vi "WAM-PROD_Sequencer.vi"() -> ()   [LabVIEW 2018]
uses:
  <vilib>/Utility/miscctls.llb/LVPositionTypeDef.ctl
  <vilib>/Utility/miscctls.llb/LVPointTypeDef.ctl
  Labview Utilities/Load and Save Controls_LV2009/RWC_Actions.ctl
  Initialize References/Sequence Globals.vi
  Infrastructure/Test Parameter Globals_1.0.0.vi
  Automated Tests/Tetra WAM/Tetra_Globals.vi
  Infrastructure/Test Result File Name Global.vi
  Initialize References/Station References Global.vi
  <vilib>/Utility/file.llb/Read Delimited Spreadsheet (string).vi
  <vilib>/Utility/file.llb/Write Delimited Spreadsheet (string).vi
panel:
  out "Results Archive File (Location on server)":path=path "C:/RageATE Results/REV-C_P-WAM_TX-ATTEN/2_12_2025/REV-C_P-WAM_TX-ATTEN_SN_WAM-000442_2309_021225-161452.csv" caption="Results Archive File \n(Location on server)"
  out "Seq Start Time":string
  out "Seq End Time":string
  out "Total Test Time":string="0.000"
  in  "User Prompt for SN (T)":bool=TRUE
  out "App Path":string="<dev mode>"
  out "FirstCall(t)":bool
  out "Inst_vi":path=path "C:/RageATE/Automated Tests/Tetra WAM/PRODUCTION/prod test vis/Tetra_PROD_Instruments.vi"
  out "Eng_NumTests":bool[](array[boolean])=[TRUE, TRUE, TRUE, TRUE, TRUE, TRUE, TRUE, TRUE]
  out "vis to run":path[](array[path])=[path "C:/RageATE/Automated Tests/Tetra WAM/PRODUCTION/prod test vis/Tetra_PROD_Instruments.vi", path "C:/RageATE/Infrastructure/GetLoopParameters_16.0.0.0.vi", path "C:/RageATE/Infrastructure/SystemTestIterator_4.3.0.0.vi", path "", path "", path "", path "", path ""]
  out "run?":bool=TRUE
  out "Stop Testing":bool
  out "Array":string[](array[string])=["C:\\RageATE\\Automated Tests\\Tetra WAM\\PRODUCTION\\prod test vis\\Tetra_PROD_Instruments.vi", "C:\\RageATE\\Infrastructure\\GetLoopParameters_16.0.0.0.vi", "C:\\RageATE\\Infrastructure\\SystemTestIterator_4.3.0.0.vi", "", "", "", "", ""]
  out "VI Name":string="WAM-PROD_Sequencer3.vi"
  out "VI Path":path=path "C:/RageATE/Projects/WAM"
  out "db_out_str":string="REV-C_TETRA_TX-ATTEN database id: 5875\r\nMoved REV-C_TETRA_TX-ATTEN_SN_WAM-000412_2248_030323-101631.csv to Synology Drive\r\nSUCCESS\r\nREV-C_TETRA_TX-PROD database id: 5876\r\nMoved REV-C_TETRA_TX-PROD_SN_WAM-000412_2248_030323-101718.csv to Synology Drive\r\nSUCCESS\r\nMoved REV-C_TETRA_RX-PROD_SN_WAM-000412_2248_030323-103734_RxCaptureFiles.zip to Synology Drive\r\nREV-C_TETRA_RX-PROD database id: 5877\r\nMoved REV-C_TETRA_RX-PROD_SN_WAM-000412_2248_030323-103734.csv to Synology Drive\r\nSUCCESS\r\nMoved WAM-C_BOUNCE_SN_WAM-000412_2248_030323-111048_Iq.csv to Synology Drive\r\nWAM-C_BOUNCE database id: 1300\r\nMoved WAM-C_BOUNCE_SN_WAM-000412_2248_030323-111048.csv to Synology Drive\r\nSUCCESS\r\n"
  out "syn_error?(t)":bool
  out "ID":string[](array[string])=["5875", "5876", "5877", "1300"]
  out "UserBCPopup_ref_out":refnum<vi>
  out "user_vi_ref":refnum<vi>
  out "EmpID(str)":string
  in  "LogFilePath":path=path "C:/RageATE Results"
  out "ABORT AT SN SCAN(T)":bool caption="OK"
  out "pw":string="RaGE_062218!"
  out "TestsArray":path[](array[path])=[path "C:/Users/ThomasWattson/OneDrive - Rage Systems/Documents - Tetra/Test Docs/Test Results/PWAM/Test Files/P-WAM-C_TX-ATTEN_Parameters.tst", path "C:/Users/ThomasWattson/OneDrive - Rage Systems/Documents - Tetra/Test Docs/Test Results/PWAM/Test Files/P-WAM-C_RX-PROD_Parameters.tst", path "C:/Users/ThomasWattson/OneDrive - Rage Systems/Documents - Tetra/Test Docs/Test Results/PWAM/Test Files/P-WAM-C_BOUNCE.tst", path "C:/Users/ThomasWattson/OneDrive - Rage Systems/Documents - Tetra/Test Docs/Test Results/PWAM/Test Files/P-WAM-C_TX-PROD_10MHZ_Parameters.tst"]
  out "result files array":path[](array[path])
  out "viRefs":refnum<vi>[](array[refnum])
  out "TestBench_ID":string="WAM_PROD_TEST-1"
  out "current time":timestamp=timestamp(3822239814.3112698 s since 1904-01-01)
  out "Array Element.Value":variant=variant(bool TRUE)
  out "TestResultLink":string="C:\\RageATE Results\\REV-C_P-WAM_TX-ATTEN\\2_12_2025\\REV-C_P-WAM_TX-ATTEN_SN_WAM-000442_2309_021225-161452.csv"
  out "BarCodeInfo":string="#RaGE Systems\r\n#Prod_Name: Wideband Antenna Module\r\n#Rage_PN: 5083561\r\n#Revision: C.08\r\n#LotID: 2309\r\n#MSN: WAM-000442\r\n#ESN: 0x00003A0E2EA5\r\n"
  in  "TabControl":T1(tab)
  in  "Load Tests":bool
  out "FileVersion":string="<dev mode>"
  out "LegalCopyright":string="<dev mode>"
  out "FileDescription":string="<dev mode>"
  out "SW Build":string="<dev mode>"
  in  "SILENCE SAFETY BUZZER":bool
  out "PostProcessMesssage":string
  in  "Test Resolution":bool=TRUE
  in  "Run All Tests (T)":bool=TRUE caption="Place entry into test log"
  in  "Run WAM BOUNCE (T)":bool=TRUE caption="Place entry into test log"
  in  "Run WAM RX (T)":bool=TRUE caption="Place entry into test log"
  in  "Run WAM TX (T)":bool=TRUE caption="Place entry into test log"
  in  "Run WAM-C Atten (t)":bool=TRUE caption="Place entry into test log"
  in  "START TESTING":bool
  out "Test Run 2":string="!!! CHECK EMPLOYEE ID BADGE! ,  Press START to Begin Testing" caption="Running Test: C:\\RageATE\\Automated Tests\\Tetra WAM\\DVT\\Tetra_RX-DVT_Parameters-Quick.tst 1 of 50"
  in  "STOP TESTING":bool
  out "PASS":bool=TRUE
  out "-ssid":string="02122025160254"
  in  "Require System Standard (T)":bool=TRUE caption="BarCoded SN Entry"
  in  "Run Final Test Result":bool=TRUE
  in  "WAM_Bar_Code_Read":bool=TRUE caption="BarCoded SN Entry"
  out "Stop Sequencer":bool
  out "Test Results File Name (Local computer,Automatically generated)":path=path "C:/RageATE Results/REV-C_P-WAM_TX-ATTEN/2_12_2025/REV-C_P-WAM_TX-ATTEN_SN_WAM-000442_2309_021225-161452.csv"
  in  "Open output file\n when test done":bool caption="Open result file automatically upon completion of each test"
  in  "PLace a result file\n copy on server(T)":bool caption="Put a copy of the result file on the server"
  in  "Recipient Email Address (use; to separate addresses)":string="rickq@ragesystems.com"
  in  "Send email notification":bool caption="Send email notification when each test is completed"
  in  "Send as attachment":bool caption="Send result file as an email attachment (if unchecked the location of the result file will be sent)"
  in  "Generate a log file entry for this test":bool=TRUE caption="Place entry into test log"
  in  "Tests Path_Eng":path[](array[path])=[path "C:/RageATE-Tetra/Automated Tests/Tetra WAM/PRODUCTION/setup files/WAM-LC_TX_Parameters -FoilTopCover.tst", path "C:/RageATE-Tetra/Automated Tests/Tetra WAM/PRODUCTION/setup files/WAM-LC_TX_BPF-1_Parameters.tst", path "C:/Users/ThomasWattson/OneDrive - Rage Systems/Documents - Tetra/Test Docs/Test Results/PWAM/Test Files/P-WAM-C_BOUNCE.tst", path "C:/Users/ThomasWattson/OneDrive - Rage Systems/Documents - Tetra/Test Docs/Test Results/PWAM/Test Files/P-WAM-C_TX-PROD_10MHZ_Parameters.tst", path "C:/RageATE/Automated Tests/Tetra WAM/PRODUCTION/setup files/WAM-C_TX-PROD_Parameters.tst", path "C:/RageATE/Automated Tests/Tetra WAM/PRODUCTION/setup files/WAM-C_RX-PROD_Parameters.tst", path "C:/RageATE/Automated Tests/Tetra WAM/PRODUCTION/setup files/WAM-C_TX-PROD-SYS-STD_Parameters.tst", path "C:/RageATE/Automated Tests/Tetra WAM/PRODUCTION/setup files/WAM-C_RX-PROD-SYS-STD_Parameters.tst"] caption="You can run uo to 8 tests in sequence   RageAte Test Parameter files ONLY !\nRun The following Tests: (Browse for file by selecting the folder to the left of the control) or drag from explorer window."
  in  "Use TAIL(t)":bool caption="Place entry into test log"
  in  "Test Count":i32[](array[numeric])=[1, 1, 1, 1, 0, 0]
  out "Test Run":string="Starting Sequencer..." caption="Running Test: C:\\RageATE\\Automated Tests\\Tetra WAM\\DVT\\Tetra_RX-DVT_Parameters-Quick.tst 1 of 50"
  in  "EmpBarCodeRead":bool=TRUE
  in  "Send to Synology Drive":bool=TRUE
  in  "Build rev suffix":string
  in  "Place entry into DB log":bool=TRUE
  in  "Prod_Mode(T)":bool=TRUE caption="Place entry into test log"
  in  "Save Eng Tests":bool caption="Save Tests"
  in  "SYSTEM STANDARD S/N":u16(ring) items=["WAM-000102", "WAM-000104"]
  in  "Tests Path_Prod":path[](array[path])=[path "C:/RageATE-Tetra/Automated Tests/Tetra WAM/PRODUCTION/setup files/WAM-C_TX-ATTEN_Parameters.tst", path "C:/RageATE-Tetra/Automated Tests/Tetra WAM/PRODUCTION/setup files/WAM-C_BOUNCE.tst", path "C:/RageATE-Tetra/Automated Tests/Tetra WAM/PRODUCTION/setup files/WAM-C_TX-PROD-250M_Parameters.tst", path "C:/RageATE-Tetra/Automated Tests/Tetra WAM/PRODUCTION/setup files/WAM-C_RX-PROD-250M_Parameters.tst", path "C:/RageATE-Tetra/Automated Tests/Tetra WAM/PRODUCTION/setup files/WAM-C_TX-PROD_Parameters.tst", path "C:/RageATE-Tetra/Automated Tests/Tetra WAM/PRODUCTION/setup files/WAM-C_RX-PROD_Parameters.tst", path "C:/RageATE-Tetra/Automated Tests/Tetra WAM/PRODUCTION/setup files/WAM-C_TX-PROD-SYS-STD_Parameters.tst", path "C:/RageATE-Tetra/Automated Tests/Tetra WAM/PRODUCTION/setup files/WAM-C_RX-PROD-SYS-STD_Parameters.tst"] caption="WAMC Production Test Files"
  out "AppSupportPath":path=path "C:/Program Files (x86)/National Instruments/LabVIEW 2018/SupportFiles"
  out "AppSupportPath 2":path=path "C:/Program Files (x86)/National Instruments/LabVIEW 2018/SupportFiles_2"
  out "AppSupportPath 3":path=path "C:/Program Files (x86)/National Instruments/LabVIEW 2018/SupportFiles_3"
  out "IsRuntime?":bool
  out "App path":path=path "C:/Program Files (x86)/National Instruments"
  out "App Name":string="LabVIEW.exe"
  out "Application:Directory Path":path
  out "ctrl file path":path
  in  "Save Prod Tests":bool caption="Save Tests"
  out "Dev_Supportpath":path
  out "REV-C?(T)":bool
  out "logfileout":string="C:\\RageATE Results\\RageAte_Test Log_0225.csv"
  in  "Enable S11 Cal(t)":bool=TRUE caption="BarCoded SN Entry"
  in  "Results Parent Dir":path=path "C:/RageATE-Tetra Results"
  in  "Instrument File":path=path "C:/RageATE-Tetra/Automated Tests/Tetra WAM/PRODUCTION/Test Benches/Common/WAM_PROD_TEST_Instruments.csv" caption="Test Parameters File"
  in  "SendGantryHome(t)":bool
  in  "Use Serial log(T)":bool caption="Boolean 9"
  in  "Ser log Folder":path=path "C:/RageATE Results/Serial Logs" caption="Test Parameters File"
  in  "RunS11CalCheck(T)":bool=TRUE caption="BarCoded SN Entry"
  in  "HrsToFlag":dbl=72.0 format="%#_13g"
  in  "Force an S11 Cal(T)":bool caption="BarCoded SN Entry"
  in  "Use Admin Mode(T)":bool caption="Place entry into test log"
  in  "Bypass EmpBarCodeRead":bool
  out "cancelled(t)":bool
  out "EMPID_OK?(t)":bool caption="OK"
  out "S11_Success(t)":bool caption="OK"
  in  "Vi Sequence":T2={"Vis to run in sequence"=[path "C:/RageATE/Automated Tests/Tetra WAM/PRODUCTION/prod test vis/Tetra_PROD_Instruments.vi", path "C:/RageATE-Tetra/Infrastructure/GetLoopParameters.vi", path "C:/RageATE-Tetra/Infrastructure/SystemTestIterator.vi", path "", path "", path "", path "", path ""], "Run"=[TRUE, TRUE, TRUE, FALSE, FALSE, FALSE, FALSE, FALSE], "Panel Behavior"=[1, 1, 1, 1, 1, 3, 1, 1], "Close Panel(T)"=[TRUE, TRUE, TRUE, FALSE, FALSE, FALSE, FALSE, FALSE]} {"Panel Behavior" items=["Invalid", "Standard", "Closed", "Hidden", "Minimized", "Maximized"]}
  in  "Save Vi Sequence":bool
  in  "force_lc(t)":bool
  in  "Create a System Standard":bool
  in  "Launch Post Processer GUI":bool
  in  "Launch Tetra Lab GUI":bool
  in  "Launch Switch GUI":bool
  in  "Launch Power Supply GUI":bool
  in  "LaunchFieldTestApp":bool
  in  "Launch Gantry App":bool
  in  "Perform a Factory Calibration":bool
  in  "error in":errorcluster
  out "More than 1 test?(T)":bool=TRUE
  out "size(s)":i32=4
  out "error out":errorcluster={"status"=TRUE, "code"=7, "source"="Open VI Reference in WAM-PROD_Sequencer.vi<APPEND>\nVI Path: <b></b>"}
  out "Close errors":errorcluster[](array[cluster])=[{"status"=FALSE, "code"=0, "source"=""}, {"status"=FALSE, "code"=0, "source"=""}, {"status"=TRUE, "code"=1039, "source"="Invoke Node in Open vi Reference_2.2.0.0.vi:7490001->WAM-PROD_Sequencer3.vi\n<APPEND>\nVI was aborted"}, {"status"=FALSE, "code"=0, "source"=""}, {"status"=FALSE, "code"=0, "source"=""}, {"status"=FALSE, "code"=0, "source"=""}, {"status"=FALSE, "code"=0, "source"=""}, {"status"=FALSE, "code"=0, "source"=""}]
  # "file:///C:\\RageATE%20Results\\WAM-C_BOUNCE\\11_3_2023\\WAM-C_BOUNCE_SN_WAM-000350_2242_110323-152039.csv"
  # "Test Selection (Default = Run All)"
  # "COMPLETED TEST  INFO"
  # "Sequence Status:"
  # "Test Selection - Eng Test"
  # "Test #"
  # "1\n2\n3\n4\n5\n6\n7\n8"
  # "Results Options Area"
  # "Notification Options"
  # "Rage Instrument File"
  # "Use the Buttons Here to Launch Varios Manual Tools for running the ATE Station"
  # "[Labview] Set Voltage and Current Limits, Turn Main Power ON/OFF"
  # "[Labview] Set RF Box Switch Positions"
  # "Launch Fieldtest.exe"
  # "[Labview] Gantry GUI to move Antenna Manually, Set Z and HOME"
  # "Launches Glens Famous TetraLabGUIGantry GUI"
  # "Check to See if A UNIT P/F (need txid,rxid,bid)"
  # "NOTE: Some of the tools {Labview] need to close {STOP BUTTONS] prior to continuing to test"
  # "Do a Full Factory Cal for T/R (Excludes REF PATH) --BETA VERSION"
  # "Create TX and RX Sys Standard Test - Requires Password"
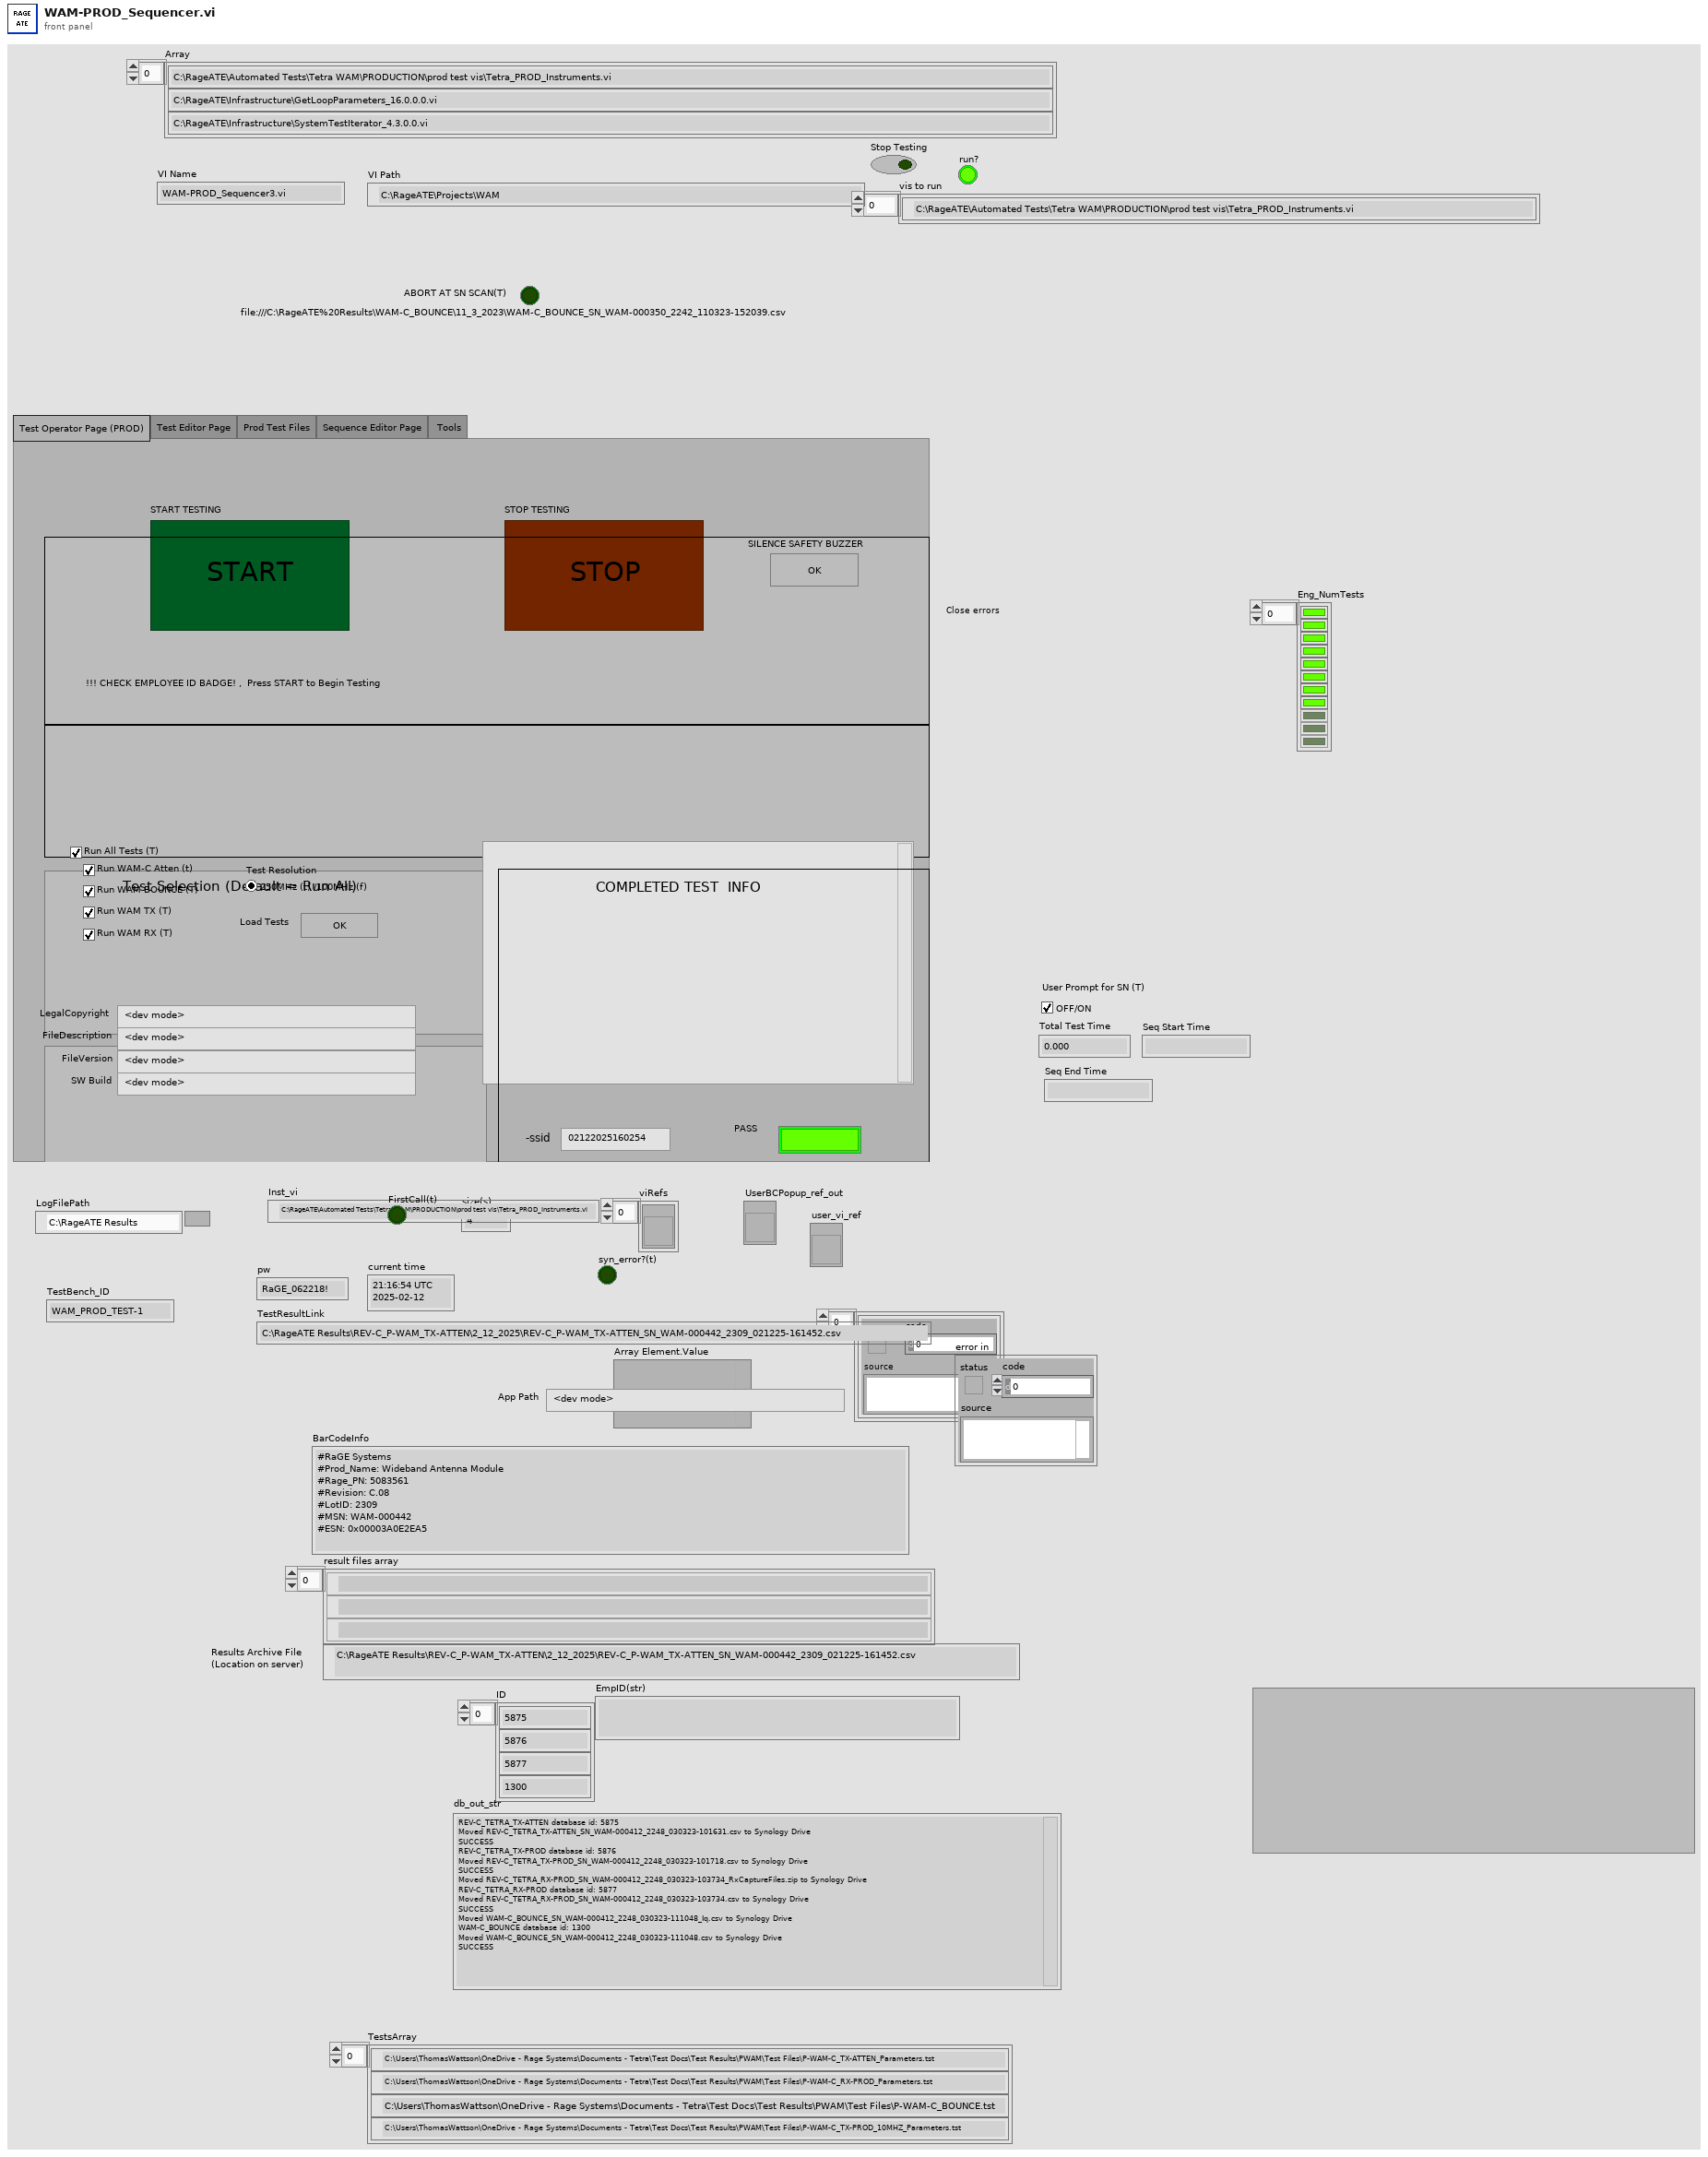
[diagram p1: front panel]
types:
  T1 = enum32{"Test Operator Page (PROD)", "Test Editor Page", "Prod Test Files", "Sequence Editor Page", " Tools"}
  T2 = cluster{"Vis to run in sequence":path[], "Run":bool[], "Panel Behavior":u16[], "Close Panel(T)":bool[]}
  T3 = typedef "RWC_Actions.ctl" = enum16{"Read", "Write", "Read and Create"}
  T4 = typedef "LVPointTypeDef.ctl" = cluster{"Horizontal":i16, "Vertical":i16}
  T5 = enum32{"Invalid", "Standard", "Closed", "Hidden", "Minimized", "Maximized"}
  T6 = enum32{"invalid app kind", "Development System", "Run Time System", "Student Edition", "Embedded LabVIEW", "Evaluation", "Custom"}
  T7 = typedef "LVPositionTypeDef.ctl" = cluster{"Left":i32, "Top":i32}
  T8 = typedef "LVRectTypeDef.ctl" = cluster{"Left":i16, "Top":i16, "Right":i16, "Bottom":i16}
  T9 = typedef "FileVersionInformation.ctl" = cluster{"FileVersion":string, "ProductName":string, "InternalName":string, "CompanyName":string, "LegalCopyright":string, "FileDescription":string}
  T10 = enum16{"open", "replace", "create", "open or create", "replace or create", "replace or create with confirmation"}
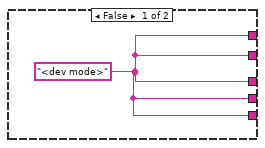
[diagram p5: hidden frame]
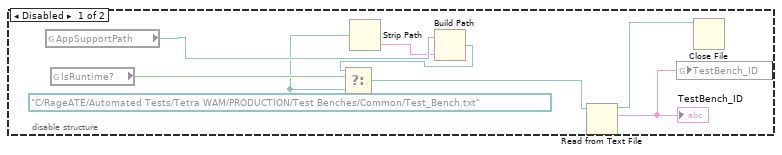
[diagram p6: hidden frame]
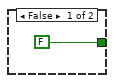
[diagram p10: hidden frame]
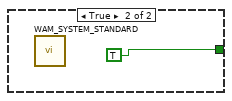
[diagram p11: hidden frame]
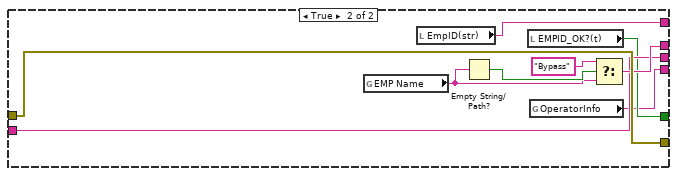
[diagram p12: hidden frame]
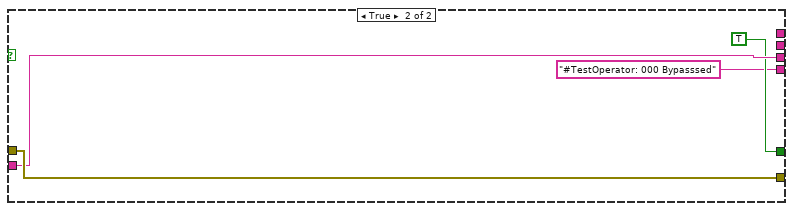
[diagram p13: hidden frame]
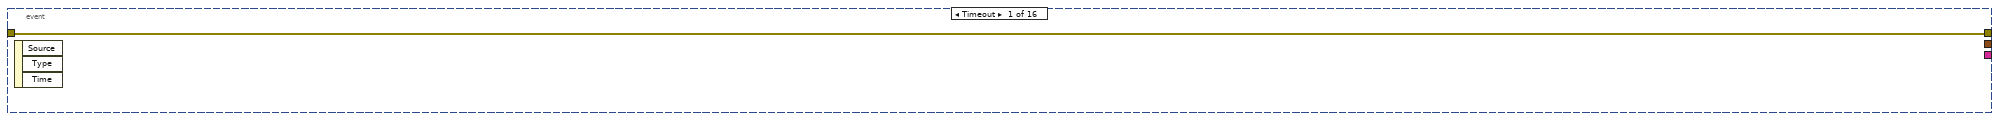
[diagram p14: hidden frame]
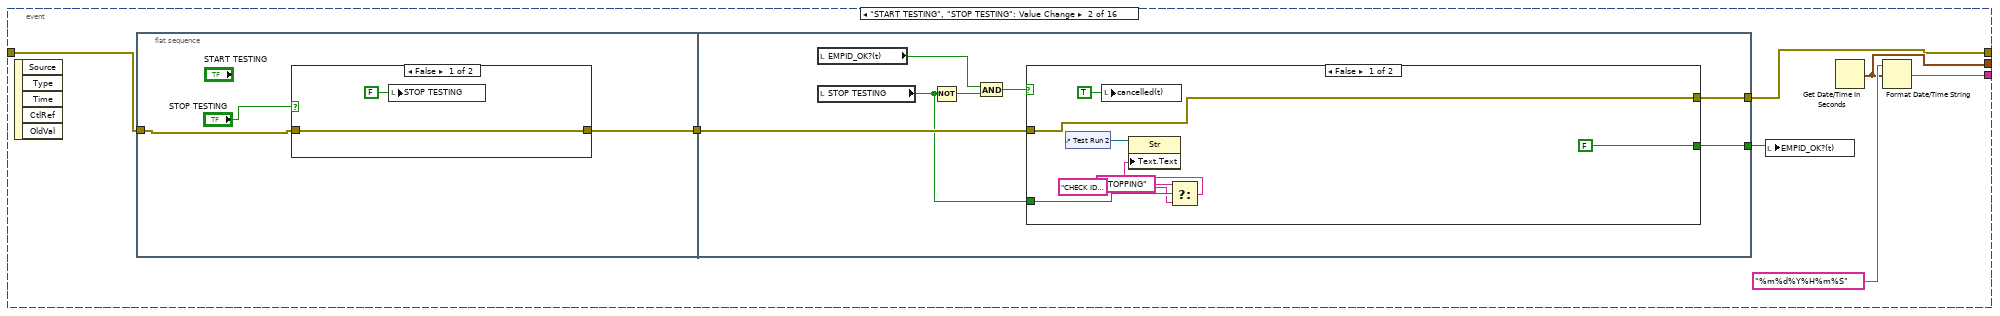
[diagram p15: hidden frame]
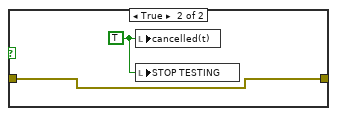
[diagram p16: hidden frame]
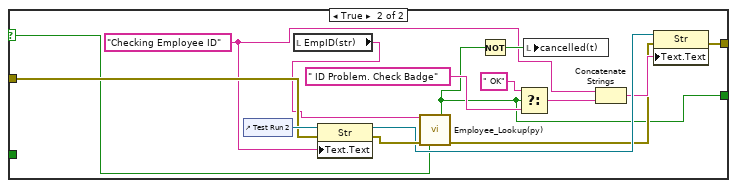
[diagram p17: hidden frame]
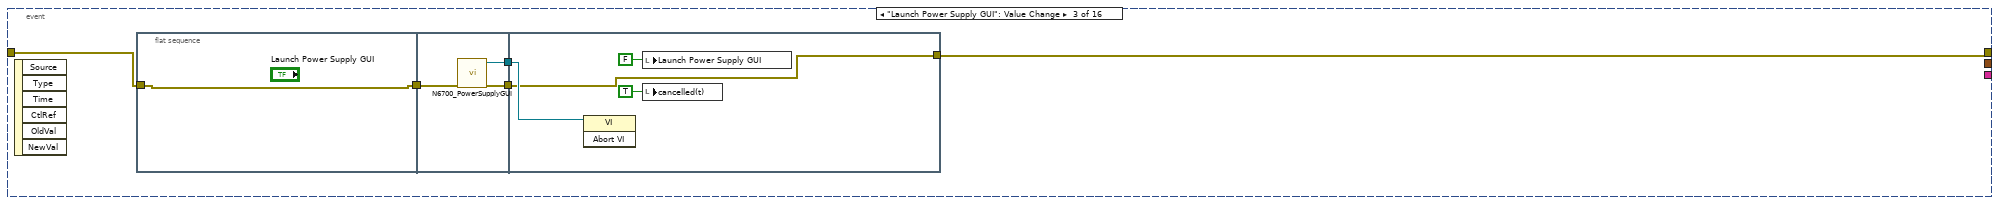
[diagram p18: hidden frame]
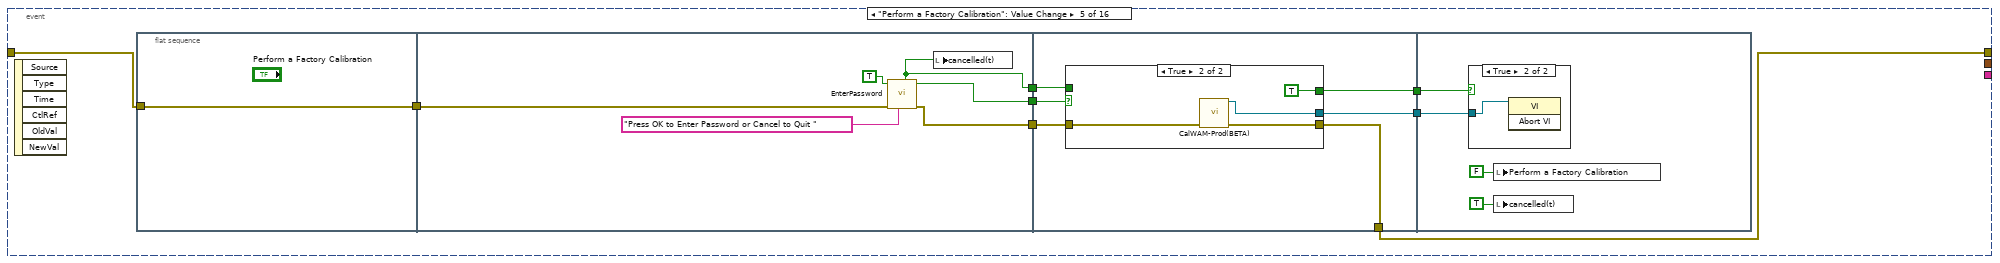
[diagram p19: hidden frame]
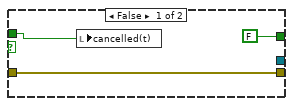
[diagram p20: hidden frame]
diagram:
  n1 = while {
    tunnel: [w11] -> w1
    stop <- w10 stop-if-true
    # "001, RICK QUIntaL, NbpT"
    # "The Calibration was Successful"
    n2 = First Call?() -> (First Call?: T/F=w3:bool)
    "FirstCall(t)" <- w3
    n3 = global write "Station References Global.vi" "Run Cal Popup"(w3) -> ()
    n4 = flat-sequence {
      tunnel: ["error in"] -> w21
      tunnel: ["Run Final Test Result"] -> w20
      tunnel: w21 -> [w158]
      tunnel: [w158] -> w19
      tunnel: w20 -> [w160]
      tunnel: [w175] -> w18
      tunnel: w19 -> [w174]
      tunnel: [w247] -> w4
      tunnel: w18 -> [w246]
      tunnel: [w659] -> w17
      tunnel: w4 -> [w659]
      tunnel: [w662] -> w16
      tunnel: w17 -> [w664]
      tunnel: [w663] -> w15
      tunnel: w16 -> [w817]
      tunnel: [w816] -> w9
      tunnel: w15 -> [w818]
      tunnel: w9 -> [w864]
      tunnel: [w863] -> w8
      tunnel: [w861] -> w2
      tunnel: [w940] -> w14
      tunnel: w8 -> [w935]
      tunnel: w2 -> [w934]
      tunnel: [w1034] -> w13
      tunnel: w14 -> [w1033]
      tunnel: w13 -> [w1198]
      tunnel: [w1199] -> w12
      tunnel: w12 -> [w1235]
      tunnel: [w1235] -> w5
      tunnel: [w1249] -> w7
      tunnel: [w1247] -> w6
      tunnel: w5 -> [w1250]
      tunnel: [w1390] -> w10
      tunnel: [w1392] -> w11
      tunnel: w7 -> [w1392]
      tunnel: w6 -> [w1391]
      frame #0 {
        w44 = T6."Run Time System"  # y
        n5 = Open Application Reference() -> (3:w45:refnum<vi>)  [unwired: 4 in, 1 out]
        n6 = control-ref of="This VI"() -> (w47:refnum<vi>)
        n7 = property class="App"(reference=w45) -> (reference out=w48:refnum<vi>, "App.Kind"=w46:T6, "App.Name"=w42:string)  [unwired: 1 in, 1 out]
        "App Name" <- w42
        n8 = flat-sequence {
          frame #0 {
            n9 = disable-structure shown="Disabled" {
              frame Disabled {
                w97 = TRUE  # Activate?
                w96 = T5."Standard"  # State
                n10 = property class="VI" props=["FP.State"]() -> (error out=w98:errorcluster)  [unwired: 2 in, 2 out]
                n11 = invoke class="VI" method="FP.Open"(error in=w98, "Activate"=w97, "State"=w96) -> ()  [unwired: 2 in, 5 out]
              }
              frame Enabled {
              }
            }
            n12 = flat-sequence {
              frame #0 {
                w71 = FALSE ("Front Panel Window:Resizable")
                w92 = T7 {"Left"=0, "Top"=0}  # Position
                # "Read the size and location of tab and size the window to it"
                n13 = property class="VI"() -> ("Front Panel Window:Open"=w70:bool)  [unwired: 2 in, 2 out]
                n14 = control-ref of="This VI"() -> (w72:refnum<vi>)
                n15 = property class="VI"(reference=w72, "Front Panel.Resizeable"=w71, "Front Panel.ShowMenuBar"=w71) -> ()  [unwired: 1 in, 2 out]
                n16 = property class="VI"(reference=w72) -> ("Panel"=w73:refnum<vi>)  [unwired: 1 in, 2 out]
                n17 = case shown="False" w70 {
                  frame False {
                    n18 = property class="VI"("Front Panel Window:Open"=TRUE) -> ()  [unwired: 2 in, 2 out]
                  }
                  frame True {
                  }
                }
                n19 = property class="Pnl"(reference=w73) -> ("Panes[]"=w76:refnum<vi>[])  [unwired: 1 in, 2 out]
                n20 = Index Array(array=w76) -> (element=w75:refnum<vi>)  [unwired: 1 in]
                n21 = property class="Pane"(reference=w75, "Origin"=T4 {"Horizontal"=0, "Vertical"=0}) -> (reference out=w90:refnum<vi>, error out=w81:errorcluster)  [unwired: 1 in]
                n22 = property class="Pane"(reference=w90, error in=w81) -> ("Origin"=w93:T4)  [unwired: 2 out]
                n23 = Unbundle By Name(w93) -> ("Horizontal"=w94:i16, "Vertical"=w91:i16)
                n24 = control-ref of="This VI"() -> (w88:refnum<vi>)
                n25 = control-ref of="TabControl"() -> (w74:refnum<vi>)
                n26 = property class="VI"(reference=w88) -> (error out=w80:errorcluster, "Front Panel.PanelBounds"=w82:T8)  [unwired: 1 in, 1 out]
                n27 = Bundle By Name(cluster=w92, "Left"=w94, "Top"=w91) -> (w79:T7)
                n28 = property class="TabCtl (strict)"(reference=w74, "Position"=w79) -> ("Height"=w78:u32, "Width"=w77:u32)  [unwired: 1 in, 2 out]
                n29 = Unbundle By Name(w82) -> ("Top"=w87:i16, "Left"=w84:i16)  [unwired: 2 out]
                n30 = Add(x=w78, y=w87) -> (x+y=w85:u32)
                n31 = Add(x=w84, y=w77) -> (x+y=w83:u32)
                n32 = Bundle By Name(cluster=w82, "Top"=w87, "Bottom"=w85, "Left"=w84, "Right"=w83) -> (w86:T8)
                n33 = property class="VI"(error in=w80, "Front Panel.PanelBounds"=w86) -> ()  [unwired: 1 in, 2 out]
              }
            }
          }
        }
        n34 = property class="VI" props=["Path", "VIType"](reference=w47) -> ("Path"=w40:path)  [unwired: 1 in, 3 out]
        n35 = property class="App"(reference=w48) -> ("App.Dir"=w22:path)  [unwired: 1 in, 2 out]
        "Application:Directory Path" <- w22
        n36 = call <vilib>:"Application Directory.vi"() -> ("Application Directory"=w43:path)
        n37 = Strip Path(path=w40) -> (stripped path=w32:path, name=→"VI Name":string)
        "VI Path" <- w32
        n38 = Equal?(x=w46, y=w44) -> (x = y?=w25:bool)
        "IsRuntime?" <- w25
        n39 = Build Path(base path=w43, name or relative path=w42) -> (appended path=w36:path)
        n40 = Strip Path(path=w22) -> (stripped path=→"App path":path)  [unwired: 1 out]
        n41 = global write "Sequence Globals.vi" "IsRuntime?"(w25) -> ()
        n42 = Strip Path(path=w32) -> (stripped path=w31:path)  [unwired: 1 out]
        n43 = case shown="True" w25 {
          tunnel: [w99 w114] -> w41
          tunnel: [w99 w112] -> w39
          tunnel: [w99 w111] -> w38
          tunnel: [w99 w110] -> w37
          tunnel: w36 -> [_ w109]
          tunnel: [_ w105] -> w35
          tunnel: [_ w104] -> w34
          tunnel: [_ w103] -> w33
          tunnel: w22 -> [_ w102]
          tunnel: [w99 w100] -> w28
          frame False {
            w99 = "<dev mode>" ("File Version Info")
          }
          frame True {
            w108 = "SupportFiles_3"  # name or relative path
            w107 = "SupportFiles_2"  # name or relative path
            w106 = "SupportFiles"  # name or relative path
            n44 = call "FileVersionInfo.vi"("Application Path in"=w109) -> ("FileVersionInfo Out"=w113:T9, "File Version Info"=w114:string, "Application Path out"=w101:path)  [unwired: 7 in, 1 out]
            n45 = Unbundle By Name(w113) -> ("FileVersion"=w112:string, "LegalCopyright"=w111:string, "FileDescription"=w110:string)
            n46 = Path To String(path=w101) -> (string=w100:string)
            n47 = Build Path(base path=w102, name or relative path=w106) -> (appended path=w103:path)
            n48 = Build Path(base path=w102, name or relative path=w108) -> (appended path=w105:path)
            n49 = Build Path(base path=w102, name or relative path=w107) -> (appended path=w104:path)
          }
        }
        "AppSupportPath" <- w33
        "AppSupportPath 2" <- w34
        "AppSupportPath 3" <- w35
        "SW Build" <- w41
        "FileVersion" <- w39
        "LegalCopyright" <- w38
        "FileDescription" <- w37
        "App Path" <- w28
        n50 = Strip Path(path=w31) -> (stripped path=w30:path)  [unwired: 1 out]
        n51 = Build Path(base path=w30, name or relative path="Support") -> (appended path=w27:path)
        "Dev_Supportpath" <- w27
        n52 = global write "Sequence Globals.vi" "DevSupportPath"(w27) -> ()
        n53 = global write "Sequence Globals.vi" "AppSupportPath"(w33) -> ()
        n54 = global write "Sequence Globals.vi" "AppSupportPath 3"(w35) -> ()
        n55 = global write "Sequence Globals.vi" "AppSupportPath 2"(w34) -> ()
        n56 = Select(t=w22, s=w25, f=w27) -> (s? t:f=w23:path)
        "ctrl file path" <- w23
        n57 = First Call?() -> (First Call?: T/F=w24:bool)
        n58 = case shown="True" w24 {
          tunnel: w23 -> [_ w54]
          frame False {
          }
          frame True {
            n59 = control-ref of="Vi Sequence"() -> (w59:refnum<vi>)
            n60 = control-ref of="Test Count"() -> (w53:refnum<vi>)
            n61 = control-ref of="Tests Path_Eng"() -> (w69:refnum<vi>)
            n62 = control-ref of="Tests Path_Prod"() -> (w65:refnum<vi>)
            n63 = Build Array(w53) -> (w57:refnum<vi>[])
            n64 = Build Array(w69) -> (w62:refnum<vi>[])
            n65 = Build Array(w59) -> (w58:refnum<vi>[])
            n66 = Build Array(w65) -> (w68:refnum<vi>[])
            n67 = call "Read and Write Controls to Automatic Config File.vi"("path"=w54, "Use Path"=TRUE ("Use vi Path"), "Action"=RWC_Actions."Read", "Control References"=w68) -> ("error out"=w52:errorcluster)  [unwired: 6 in, 1 out]
            n68 = call "Read and Write Controls to Automatic Config File.vi"("path"=w54, "Use Path"=TRUE ("Use vi Path"), "Action"=RWC_Actions."Read", "error in"=w52, "Control References"=w62) -> ("error out"=w51:errorcluster)  [unwired: 5 in, 1 out]
            n69 = call "Read and Write Controls to Automatic Config File.vi"("path"=w54, "Use Path"=TRUE ("Use vi Path"), "Action"=RWC_Actions."Read", "error in"=w51, "Control References"=w57) -> ("error out"=w50:errorcluster)  [unwired: 5 in, 1 out]
            n70 = call "Read and Write Controls to Automatic Config File.vi"("path"=w54, "Use Path"=TRUE ("Use vi Path"), "Action"=RWC_Actions."Read", "error in"=w50, "Control References"=w58) -> ()  [unwired: 5 in, 2 out]
          }
        }
      }
      frame #1 {
        w115 = string[] ["2.6.1*", "<error>*", "<error>*", "<error>*", "<error>*", "1.0.4*"]  # Ver_Tags(ary)
        w116 = "#Gitlog Commit: ea2f676a6d19232e7cb3d3269445d2cde244cf19   Ver: 2.6.1\n#Gitlog Author: Rick-Rage <74794943+Rick-Rage@users.noreply.github.com>\n#Gitlog Date:   Tue Jan 9 15:17:04 2024 -0500\n#Gitlog ComputerName: OMAHA"  # RageATE_Gitlog
        w117 = T1."Test Operator Page (PROD)"  # TabControl
        w125 = FALSE ("START TESTING")
        n71 = control-ref of="Run"() -> (w128:refnum<vi>)
        n72 = flat-sequence {
          frame #0 {
            w150 = ""
            w149 = FALSE ("Stop Sequencer")
            n73 = First Call?() -> (First Call?: T/F=w146:bool)
            n74 = local write "Seq End Time"(w150) -> ()
            n75 = local write "Seq Start Time"(w150) -> ()
            n76 = case shown="True" w146 {
              frame False {
              }
              frame True {
                "EMPID_OK?(t)" <- FALSE ("EMPID_OK?(t)")
              }
            }
            n77 = global write "Test Parameter Globals_1.0.0.vi" "Use TAIL"("Use TAIL(t)") -> ()
            n78 = local read "Tests Path_Eng"() -> (w147:path[])
            n79 = for {
              tunnel: w147 -> [w156] mode=indexing
              tunnel: [w154] -> w148 mode=indexing
              n80 = Empty String/Path?(string/path=w156) -> (empty?=w155:bool)
              n81 = Not(x=w155) -> (.not. x?=w154:bool)
            }
            "Eng_NumTests" <- w148
            n82 = global write "Test Result File Name Global.vi" "Results Parent Dir"("Results Parent Dir") -> ()
            n83 = local write "LogFilePath"("Results Parent Dir") -> ()
            "pw" <- "RaGE_062218!" ("pw")
            "Stop Sequencer" <- w149
            "cancelled(t)" <- w149
          }
        }
        n84 = First Call?() -> (First Call?: T/F=w124:bool)
        n85 = property class="Arr (strict)"(reference=w128) -> ("Array Element.Value"=w129:variant)  [unwired: 1 in, 2 out]
        "Array Element.Value" <- w129
        n86 = case shown="True" w124 {
          tunnel: w125 -> [_ w157]
          frame False {
          }
          frame True {
            "ABORT AT SN SCAN(T)" <- w157
          }
        }
        n87 = local write "START TESTING"(w125) -> ()
        n88 = global write "Sequence Globals.vi" "Stop Testing"(w125) -> ()
        n89 = local write "STOP TESTING"(w125) -> ()
        n90 = global write "Test Parameter Globals_1.0.0.vi" "Setup.vi Error"(errorcluster {"status"=FALSE, "code"=0, "source"=""} ("Setup.vi Error")) -> ()
        n91 = Not(x="Use Admin Mode(T)") -> ()  [unwired: 1 out]
        n92 = local write "Array Element.Value"(w129) -> ()
        n93 = property on="TabControl" class="TabCtl (strict)"("Value"=w117) -> (error out=w121:errorcluster)  [unwired: 2 in, 1 out]
        n94 = disable-structure shown="Enabled" {
          frame Disabled {
            w139 = path "C:/RageATE/Automated Tests/Tetra WAM/PRODUCTION/Test Benches/Common/Test_Bench.txt" ("file (use dialog)")
            n95 = global read "Sequence Globals.vi" "AppSupportPath"() -> (w142:path)
            n96 = global read "Sequence Globals.vi" "IsRuntime?"() -> (w140:bool)
            n97 = Strip Path(path=w139) -> (name=w141:string)  [unwired: 1 out]
            n98 = Build Path(base path=w142, name or relative path=w141) -> (appended path=w137:path)
            n99 = Select(t=w137, s=w140, f=w139) -> (s? t:f=w138:path)
            n100 = Read from Text File(file (use dialog)=w138) -> (refnum out=w143:refnum<file>, text=w144:string)  [unwired: 3 in, 2 out]
            "TestBench_ID" <- w144
            n101 = global write "Tetra_Globals.vi" "TestBench_ID"(w144) -> ()
            n102 = Close File(refnum=w143) -> ()  [unwired: 1 in, 2 out]
          }
          frame Enabled {
          }
        }
        n103 = stacked-sequence {
          frame #0 {
            n104 = global read "Sequence Globals.vi" "AppSupportPath"() -> (w135:path)
            n105 = Strip Path(path="Instrument File") -> (name=w136:string)  [unwired: 1 out]
            n106 = local read "IsRuntime?"() -> (w133:bool)
            n107 = Build Path(base path=w135, name or relative path=w136) -> (appended path=w134:path)
            n108 = Select(t=w134, s=w133, f="Instrument File") -> (s? t:f=w131:path)
            n109 = global write "Sequence Globals.vi" "Inst File"(w131) -> ()
          }
        }
        n110 = property on="TabControl" class="TabCtl (strict)"(error in=w121, "PageSelVis"=TRUE ("Page Selector Visible")) -> (error out=w119:errorcluster)  [unwired: 1 in, 1 out]
        n111 = control-ref of="Test Run 2"() -> (w123:refnum<vi>)
        n112 = property class="Str"(reference=w123, error in=w119, "Text.Text"="Starting Sequencer...") -> ()  [unwired: 2 out]
        n113 = global write "Sequence Globals.vi" "RageATE_Gitlog"(w116) -> ()
        n114 = global write "Sequence Globals.vi" "Gitlog"(w116) -> ()
        n115 = global write "Tetra_Globals.vi" "Ver_Tags(ary)"(w115) -> ()
      }
      frame #2 {
        w159 = FALSE  # stop? (T)
        n116 = local write "Send to Synology Drive"(w160) -> ()
        n117 = Stop(stop? (T)=w159) -> ()
      }
      frame #3 {
        n118 = local read "EMPID_OK?(t)"() -> (w169:bool)
        n119 = global read "Tetra_Globals.vi" "PASS_SYS-STD(T)"() -> (w162:bool)
        n120 = local read "Prod_Mode(T)"() -> (w164:bool)
        n121 = local read "Require System Standard (T)"() -> (w166:bool)
        n122 = Not(x=w162) -> (.not. x?=w161:bool)
        n123 = And(x=w161, y=w164) -> (x .and. y?=w163:bool)
        n124 = And(x=w166, y=w163) -> (x .and. y?=w165:bool)
        n125 = case shown="False" "Bypass EmpBarCodeRead" {
          tunnel: [w206 w244] -> w178
          tunnel: w174 -> [w205 w244]
          tunnel: "EmpBarCodeRead" -> [w203 _]
          tunnel: [w204 "#TestOperator: 000 Bypasssed" ("OperatorInfo")] -> w177
          tunnel: [w202 _] -> w181
          tunnel: w169 -> [w201 _]
          tunnel: " ,  Press START to Begin Testing" ("Text.Text") -> [w200 w243]
          tunnel: [w199 w243] -> w171
          tunnel: [w198 TRUE ("OK")] -> w168
          tunnel: [w197 _] -> w170
          frame False {
            n126 = case shown="False" w201 {
              tunnel: [w221 w240] -> w206
              tunnel: w205 -> [w215 w240]
              tunnel: [w212 w233] -> w204
              tunnel: w203 -> [w220 _]
              tunnel: [w218 w237] -> w202
              tunnel: [w216 w235] -> w199
              tunnel: w200 -> [w217 w235]
              tunnel: [w208 w234] -> w198
              tunnel: [w207 w232] -> w197
              frame False {
                n127 = property class="VI"(error in=w215, "Front Panel.IsFrontmost"=FALSE ("Front Panel Window:Is Frontmost")) -> (error out=w214:errorcluster)  [unwired: 1 in, 1 out]
                n128 = for {
                  N: 1 -> [_]
                  tunnel: [w228] -> w211
                  tunnel: w220 -> [w229]
                  shift-right: [w231] -> w221
                  shift-left: w214 -> [w230]
                  tunnel: [w227] -> _
                  tunnel: [w226] -> w218
                  tunnel: [w225] -> w210
                  tunnel: [w225] -> w208
                  tunnel: [w224] -> w207
                  stop <- w227 continue-if-true
                  n129 = call "WAM_UserInput_Popup.vi"("error in (no error)"=w230, "UseBcScanner(t)"=w229) -> ("EmpName"=w226:string, "UserString"=w224:string, "operator infor header"=w228:string, "UserInput_Popup_refOut"=→"user_vi_ref":refnum<vi>, "UserBCPopup_ref_out"=→"UserBCPopup_ref_out":refnum<vi>, "OK"=w225:bool, "error out"=w231:errorcluster)  [unwired: 11 in]
                  n130 = Empty String/Path?(string/path=w224) -> (empty?=w227:bool)
                }
                n131 = Select(t=w211, s=w210, f="!!! CHECK EMPLOYEE ID BADGE!" ("Text.Text")) -> (s? t:f=w212:string)
                n132 = Concatenate Strings(w212, w217) -> (w216:string)
              }
              frame True {
                n133 = global read "Test Parameter Globals_1.0.0.vi" "EMP Name"() -> (w238:string)
                n134 = local read "EmpID(str)"() -> (w232:string)
                n135 = Empty String/Path?(string/path=w238) -> (empty?=w239:bool)
                n136 = local read "EMPID_OK?(t)"() -> (w234:bool)
                n137 = global read "Test Parameter Globals_1.0.0.vi" "OperatorInfo"() -> (w233:string)
                n138 = Select(t="Bypass", s=w239, f=w238) -> (s? t:f=w237:string)
              }
            }
          }
          frame True {
          }
        }
        "EmpID(str)" <- w170
        n139 = And(x=w168, y=w165) -> (x .and. y?=w167:bool)
        n140 = case shown="True" w167 {
          frame False {
          }
          frame True {
            n141 = property on="SYSTEM STANDARD S/N" class="Ring (strict)"() -> ("RingText.Text"=w186:string)  [unwired: 2 in, 2 out]
            n142 = Format Into String(format string="You Need to Run a System Standard prior to testing !! \nAttach a system Standard with the SN: %s and continue OR Exit to Quit \nIf you QUIT and Enter a Admin PW, you can go to tools tab and create a system standard ", w186) -> (resulting string=w185:string)  [unwired: 2 in, 1 out]
            n143 = Two Button Dialog(message=w185) -> (T button?=w183:bool)  [unwired: 2 in]
            n144 = Not(x=w183) -> (.not. x?=w184:bool)
            n145 = local write "cancelled(t)"(w184) -> ()
            n146 = case shown="False" w183 {
              tunnel: [w189 TRUE] -> w182
              frame False {
                n147 = call "Display Message to User6"() -> ("OK"=w188:bool)  [unwired: 10 in, 1 out]
                n148 = case shown="True" w188 {
                  selector: w188 -> [_ w191]
                  tunnel: [FALSE ("success(t)") w192] -> w189
                  frame False {
                  }
                  frame True {
                    n149 = call "EnterPassword.vi"("Enable(t)"=w191) -> ("success(t)"=w193:bool, "cancelled(t)"=w195:bool)  [unwired: 8 in, 1 out]
                    n150 = Not(x=w195) -> (.not. x?=w194:bool)
                    n151 = And(x=w194, y=w193) -> (x .and. y?=w192:bool)
                  }
                }
              }
              frame True {
                n152 = call "WAM_SYSTEM_STANDARD.vi"() -> ()  [unwired: 12 in]
              }
            }
            n153 = global write "Tetra_Globals.vi" "PASS_SYS-STD(T)"(w182) -> ()
          }
        }
        n154 = local write "EMPID_OK?(t)"(w168) -> ()
        n155 = global write "Test Parameter Globals_1.0.0.vi" "EMP Name"(w181) -> ()
        n156 = Concatenate Strings(w181, w171) -> (w180:string)
        n157 = global write "Test Parameter Globals_1.0.0.vi" "OperatorInfo"(w177) -> ()
        n158 = control-ref of="Test Run 2"() -> (w179:refnum<vi>)
        n159 = property class="Str"(reference=w179, error in=w178, "Text.Text"=w180) -> (error out=w175:errorcluster)  [unwired: 1 out]
      }
      frame #4 {
        n160 = while {
          shift-right: [w256] -> w247
          shift-left: w246 -> [w255]
          i -> [w253]
          stop <- w254 stop-if-true
          # "Cal Successful! Press OK to Continue or Repeat Cal to Repeat"
          # "The Calibration Failed or was cancelled"
          # "The Calibration was Successful"
          n161 = flat-sequence "Main Start Buttons" {
            tunnel: w255 -> [w266]
            tunnel: [w266] -> w249
            tunnel: [w268] -> w248
            tunnel: w249 -> [w267]
            tunnel: [w524] -> w252
            tunnel: w248 -> [w524]
            tunnel: [w511] -> w250
            frame #0 {
              w265 = FALSE ("STOP TESTING")
              n162 = global read "Sequence Globals.vi" "AppSupportPath"() -> (w261:path)
              n163 = local read "Vi Sequence"() -> (w257:T2)
              n164 = Unbundle By Name(w257) -> ("Vis to run in sequence"=w264:path[])
              n165 = local read "IsRuntime?"() -> (w258:bool)
              n166 = local write "STOP TESTING"(w265) -> ()
              n167 = local write "START TESTING"(w265) -> ()
              n168 = local write "Stop Sequencer"(w265) -> ()
              n169 = Index Array(array=w264) -> (element=w259:path)  [unwired: 1 in]
              n170 = Strip Path(path=w259) -> (name=w262:string)  [unwired: 1 out]
              n171 = Build Path(base path=w261, name or relative path=w262) -> (appended path=w260:path)
              n172 = Select(t=w260, s=w258, f=w259) -> (s? t:f=→"Inst_vi":path)
            }
            frame #1 {
              n173 = event shown="[3] \"Create a System Standard\": Value Change" {
                selector: _ -> [_ _ _ _ _ _ _ _ _ _ _ _ _ _ _ _]
                dyn-events: _ -> [_ _ _ _ _ _ _ _ _ _ _ _ _ _ _ _]
                timeout: -1 -> [_ _ _ _ _ _ _ _ _ _ _ _ _ _ _ _]
                tunnel: w267 -> [w276 w278 w325 _ w340 w370 w381 _ _ _ w402 w421 w446 _ w485 _]
                tunnel: [w276 w280 w321 _ w339 w369 _ _ _ _ w400 w419 w447 _ w485 _] -> w268
                tunnel: [_ w282 _ _ _ _ _ _ _ _ _ _ _ _ _ _] -> w274
                tunnel: [_ w281 _ _ _ _ _ _ _ _ _ _ _ _ _ _] -> w269
                event Timeout {
                  n174 = event-data() -> ()  [unwired: 1 in, 3 out]
                }
                event "START TESTING", "STOP TESTING": Value Change {
                  n175 = event-data() -> ()  [unwired: 1 in, 5 out]
                  n176 = flat-sequence {
                    tunnel: [w284] -> w279
                    tunnel: w278 -> [w285]
                    tunnel: [w297] -> w280
                    tunnel: w279 -> [w296]
                    tunnel: [w294] -> w277
                    frame #0 {
                      n177 = case shown="False" "STOP TESTING" {
                        tunnel: w285 -> [w287 w289]
                        tunnel: [w287 w289] -> w284
                        frame False {
                          n178 = local write "STOP TESTING"(FALSE ("STOP TESTING")) -> ()
                        }
                        frame True {
                          w290 = TRUE ("cancelled(t)")
                          n179 = local write "cancelled(t)"(w290) -> ()
                          n180 = local write "STOP TESTING"(w290) -> ()
                        }
                      }
                    }
                    frame #1 {
                      n181 = local read "EMPID_OK?(t)"() -> (w292:bool)
                      n182 = local read "STOP TESTING"() -> (w291:bool)
                      n183 = Not(x=w291) -> (.not. x?=w293:bool)
                      n184 = And(x=w292, y=w293) -> (x .and. y?=w295:bool)
                      n185 = case shown="False" w295 {
                        selector: w295 -> [_ w306]
                        tunnel: [w303 w309] -> w297
                        tunnel: w296 -> [w303 w318]
                        tunnel: [FALSE w307] -> w294
                        tunnel: w291 -> [w301 _]
                        frame False {
                          n186 = control-ref of="Test Run 2"() -> (w304:refnum<vi>)
                          n187 = local write "cancelled(t)"(TRUE ("cancelled(t)")) -> ()
                          n188 = Select(t="STOPPING", s=w301, f="CHECK ID BADGE!! STOP AND RESTART TEST" ("Text.Text")) -> (s? t:f=w299:string)
                          n189 = property class="Str"(reference=w304, "Text.Text"=w299) -> ()  [unwired: 1 in, 2 out]
                        }
                        frame True {
                          w315 = "Checking Employee ID" ("Text.Text")
                          n190 = control-ref of="Test Run 2"() -> (w319:refnum<vi>)
                          n191 = local read "EmpID(str)"() -> (w308:string)
                          n192 = property class="Str"(reference=w319, error in=w318, "Text.Text"=w315) -> (reference out=w316:refnum<vi>, error out=w317:errorcluster)
                          n193 = call "Employee_Lookup(py).vi"("Badge Scan In(str)"=w308, "error in (no error)"=w317, "Enable(t)"=w306) -> ("Success?(t)"=w307:bool, "error out"=w310:errorcluster)  [unwired: 10 in, 1 out]
                          n194 = Not(x=w307) -> (.not. x?=w320:bool)
                          n195 = Select(t=" OK" ("string"), s=w307, f=" ID Problem. Check Badge" ("string")) -> (s? t:f=w313:string)
                          n196 = local write "cancelled(t)"(w320) -> ()
                          n197 = Concatenate Strings(w315, w313) -> (w314:string)
                          n198 = property class="Str"(reference=w316, error in=w310, "Text.Text"=w314) -> (error out=w309:errorcluster)  [unwired: 1 out]
                        }
                      }
                    }
                  }
                  n199 = local write "EMPID_OK?(t)"(w277) -> ()
                  n200 = Get Date/Time In Seconds() -> (seconds since 1Jan1904=w281:timestamp)
                  n201 = Format Date/Time String(time format string (%c)="%m%d%Y%H%m%S" ("format string"), seconds (now)=w281) -> (date/time string=w282:string)  [unwired: 1 in]
                }
                event "Launch Power Supply GUI": Value Change {
                  n202 = event-data() -> ()  [unwired: 1 in, 6 out]
                  n203 = flat-sequence {
                    tunnel: w325 -> [w326]
                    tunnel: [w326] -> w324
                    tunnel: w324 -> [w329]
                    tunnel: [w328] -> w323
                    tunnel: [w327] -> w322
                    tunnel: w323 -> [w331]
                    tunnel: [w330] -> w321
                    tunnel: w322 -> [w330]
                    frame #0 {
                    }
                    frame #1 {
                      n204 = call "N6700_PowerSupplyGUI.vi"("error in (no error)"=w329) -> ("PsGuiRef"=w328:refnum<vi>, "error out"=w327:errorcluster)  [unwired: 13 in]
                    }
                    frame #2 {
                      n205 = invoke class="VI" method="Abort VI"(reference=w331) -> ()  [unwired: 2 in, 3 out]
                      n206 = local write "Launch Power Supply GUI"(FALSE ("Launch Power Supply GUI")) -> ()
                      n207 = local write "cancelled(t)"(TRUE ("cancelled(t)")) -> ()
                    }
                  }
                }
                event "Create a System Standard": Value Change {
                  w334 = FALSE ("RunS11CalCheck(T)")
                  n208 = event-data() -> ()  [unwired: 1 in, 6 out]
                  n209 = local write "Prod_Mode(T)"(w334) -> ()
                  n210 = local write "RunS11CalCheck(T)"(w334) -> ()
                  n211 = local write "Test Count"(i32[] [0, 0, 0, 0, 0, 0, 1, 1] ("Run Test\nn Times")) -> ()
                }
                event "Perform a Factory Calibration": Value Change {
                  n212 = event-data() -> ()  [unwired: 1 in, 6 out]
                  n213 = flat-sequence {
                    tunnel: [w344] -> w342
                    tunnel: w340 -> [w344]
                    tunnel: w342 -> [w349]
                    tunnel: [w348] -> w341
                    tunnel: [w346] -> w338
                    tunnel: [w345] -> w337
                    tunnel: [w356] -> w343
                    tunnel: w341 -> [w355]
                    tunnel: [w354] -> w339
                    tunnel: w338 -> [w353]
                    tunnel: w337 -> [w352]
                    tunnel: [w351] -> w336
                    tunnel: w343 -> [w365]
                    tunnel: w336 -> [w364]
                    frame #0 {
                    }
                    frame #1 {
                      n214 = call "EnterPassword.vi"("Message"="Press OK to Enter Password or Cancel to Quit ", "error in (no error)"=w349, "Enable(t)"=TRUE) -> ("error out"=w348:errorcluster, "success(t)"=w346:bool, "cancelled(t)"=w345:bool)  [unwired: 6 in]
                      n215 = local write "cancelled(t)"(w345) -> ()
                    }
                    frame #2 {
                      n216 = case shown="True" w353 {
                        tunnel: [_ w363] -> w356
                        tunnel: w355 -> [w359 w362]
                        tunnel: [w359 w361] -> w354
                        tunnel: w352 -> [w358 _]
                        tunnel: [FALSE ("cancelled(t)") TRUE ("cancelled(t)")] -> w351
                        frame False {
                          n217 = local write "cancelled(t)"(w358) -> ()
                        }
                        frame True {
                          n218 = call "CalWAM-Prod(BETA).vi"("error in (no error)"=w362) -> ("reference out"=w363:refnum<vi>, "error out"=w361:errorcluster)  [unwired: 13 in]
                        }
                      }
                    }
                    frame #3 {
                      n219 = case shown="True" w364 {
                        tunnel: w365 -> [_ w368]
                        frame False {
                        }
                        frame True {
                          n220 = invoke class="VI" method="Abort VI"(reference=w368) -> ()  [unwired: 2 in, 3 out]
                        }
                      }
                      n221 = local write "Perform a Factory Calibration"(FALSE ("Launch Power Supply GUI")) -> ()
                      n222 = local write "cancelled(t)"(TRUE ("cancelled(t)")) -> ()
                    }
                  }
                }
                event "Launch Gantry App": Value Change {
                  n223 = event-data() -> ()  [unwired: 1 in, 6 out]
                  n224 = flat-sequence {
                    tunnel: [w373] -> w371
                    tunnel: w370 -> [w373]
                    tunnel: [w374] -> w372
                    tunnel: w371 -> [w376]
                    tunnel: [w375] -> w369
                    tunnel: w372 -> [w378]
                    frame #0 {
                    }
                    frame #1 {
                      n225 = call "Gantry_GUI.vi"("COMPORT"=refnum<visa-resource-name> "COM5", "error in (no error)"=w376) -> ("GantryGuiRefOut"=w374:refnum<vi>, "error out"=w375:errorcluster)  [unwired: 15 in, 1 out]
                    }
                    frame #2 {
                      n226 = invoke class="VI" method="Abort VI"(reference=w378) -> ()  [unwired: 2 in, 3 out]
                      n227 = local write "cancelled(t)"(TRUE ("cancelled(t)")) -> ()
                      n228 = local write "Launch Gantry App"(FALSE ("Launch Power Supply GUI")) -> ()
                    }
                  }
                }
                event "SILENCE SAFETY BUZZER": Value Change {
                  n229 = event-data() -> ()  [unwired: 1 in, 6 out]
                  n230 = flat-sequence {
                    tunnel: [w383] -> w382
                    tunnel: w381 -> [w383]
                    tunnel: w382 -> [w386]
                    tunnel: [w385] -> _
                    frame #0 {
                    }
                    frame #1 {
                      w384 = u32 0 items=["OFF"=0, "RED"=1, "AMBER"=2, "GREEN"=4, "GRE+AMBER"=6, "ALL"=7, "BUZZ"=8, "RED+BUZZ"=9, "ALL+BUZZ"=15] ("Select")
                      n231 = call "RageATE-LightBar.vi"("VISA resource name"=refnum<visa-resource-name> "COM5" ("COMPORT"), "error in"=w386, "Select"=w384) -> ("error out"=w385:errorcluster)  [unwired: 10 in, 2 out]
                    }
                    frame #2 {
                      n232 = local write "SILENCE SAFETY BUZZER"(FALSE ("Launch Power Supply GUI")) -> ()
                      n233 = local write "cancelled(t)"(TRUE ("cancelled(t)")) -> ()
                    }
                  }
                }
                event Panel Close? {
                  n234 = event-data() -> ()  [unwired: 1 in, 4 out]
                  n235 = flat-sequence {
                    frame #0 {
                      n236 = global read "Tetra_Globals.vi" "comport"() -> (w392:refnum<visa-resource-name>)
                      n237 = call "CloseComAndFt.vi"("ComPort"=w392, "Skip(T)"=FALSE, "KillFT(t)"=TRUE) -> ()  [unwired: 11 in, 2 out]
                    }
                    frame #1 {
                      n238 = invoke class="VI" method="FP.Close"() -> ()  [unwired: 3 in, 3 out]
                    }
                    frame #2 {
                      n239 = invoke class="VI" method="Abort VI"() -> ()  [unwired: 3 in, 3 out]
                    }
                  }
                  n240 = event-data() -> ()  [unwired: 2 in, 1 out]
                }
                event "Launch Switch GUI": Value Change {
                  n241 = event-data() -> ()  [unwired: 1 in, 6 out]
                  n242 = flat-sequence {
                    tunnel: [w394] -> w393
                    tunnel: w393 -> [w395]
                    frame #0 {
                    }
                    frame #1 {
                      n243 = call "RfSwitch_GUI.vi"() -> ("SwitchViRef"=w394:refnum<vi>)  [unwired: 13 in, 2 out]
                    }
                    frame #2 {
                      n244 = invoke class="VI" method="Abort VI"(reference=w395) -> ()  [unwired: 2 in, 3 out]
                      n245 = local write "Launch Switch GUI"(FALSE ("Launch Switch GUI")) -> ()
                      n246 = local write "cancelled(t)"(TRUE ("cancelled(t)")) -> ()
                    }
                  }
                }
                event "Load Tests": Value Change {
                  n247 = event-data() -> ()  [unwired: 1 in, 6 out]
                  n248 = flat-sequence {
                    frame #0 {
                    }
                    frame #1 {
                    }
                    frame #2 {
                      n249 = local write "cancelled(t)"(TRUE ("cancelled(t)")) -> ()
                      n250 = local write "Load Tests"(FALSE ("Launch Switch GUI")) -> ()
                    }
                  }
                }
                event "Save Eng Tests": Value Change {
                  n251 = event-data() -> ()  [unwired: 1 in, 6 out]
                  n252 = flat-sequence {
                    tunnel: w402 -> [w404]
                    tunnel: [w404] -> w401
                    tunnel: [w410] -> w403
                    tunnel: w401 -> [w414]
                    tunnel: w403 -> [w416]
                    tunnel: [w416] -> w400
                    frame #0 {
                    }
                    frame #1 {
                      w407 = TRUE ("Use vi Path")
                      n253 = control-ref of="Test Count"() -> (w405:refnum<vi>)
                      n254 = control-ref of="Tests Path_Eng"() -> (w413:refnum<vi>)
                      n255 = local read "ctrl file path"() -> (w406:path)
                      n256 = Build Array(w413) -> (w415:refnum<vi>[])
                      n257 = Build Array(w405) -> (w408:refnum<vi>[])
                      n258 = call "Read and Write Controls to Automatic Config File.vi"("path"=w406, "Use Path"=w407, "Action"=RWC_Actions."Write", "error in"=w414, "Control References"=w415) -> ("error out"=w409:errorcluster)  [unwired: 5 in, 1 out]
                      n259 = call "Read and Write Controls to Automatic Config File.vi"("path"=w406, "Use Path"=w407, "Action"=RWC_Actions."Write", "error in"=w409, "Control References"=w408) -> ("error out"=w410:errorcluster)  [unwired: 5 in, 1 out]
                    }
                    frame #2 {
                      n260 = local write "cancelled(t)"(TRUE ("cancelled(t)")) -> ()
                      n261 = local write "Save Eng Tests"(FALSE ("Launch Switch GUI")) -> ()
                    }
                  }
                }
                event "Save Vi Sequence": Value Change {
                  n262 = event-data() -> ()  [unwired: 1 in, 6 out]
                  n263 = flat-sequence {
                    tunnel: w421 -> [w423]
                    tunnel: [w423] -> w420
                    tunnel: [w425] -> w422
                    tunnel: w420 -> [w426]
                    tunnel: w422 -> [w441]
                    tunnel: [w441] -> w419
                    frame #0 {
                    }
                    frame #1 {
                      n264 = control-ref of="Vi Sequence"() -> (w424:refnum<vi>)
                      n265 = local read "ctrl file path"() -> (w428:path)
                      n266 = Build Array(w424) -> (w429:refnum<vi>[])
                      n267 = disable-structure shown="Enabled" {
                        disable-tunnel: w429 -> [w434 w440]
                        disable-tunnel: w428 -> [w433 w435]
                        disable-tunnel: TRUE ("Use vi Path") -> [w432 w436]
                        disable-tunnel: w426 -> [w431 w438]
                        disable-tunnel: [w430 w437] -> w425
                        frame Disabled {
                          n268 = call "Load and Save Controls.vi"("path"=w433, "Use vi Path"=w432, "error in (no error)"=w431, "Control References"=w434) -> ("error out"=w430:errorcluster)  [unwired: 7 in]
                        }
                        frame Enabled {
                          n269 = call "Read and Write Controls to Automatic Config File.vi"("path"=w435, "Use Path"=w436, "Action"=RWC_Actions."Write", "error in"=w438, "Control References"=w440) -> ("error out"=w437:errorcluster)  [unwired: 5 in, 1 out]
                        }
                      }
                    }
                    frame #2 {
                      n270 = local write "cancelled(t)"(TRUE ("cancelled(t)")) -> ()
                      n271 = local write "Save Vi Sequence"(FALSE ("Launch Switch GUI")) -> ()
                    }
                  }
                }
                event "Save Prod Tests": Value Change {
                  n272 = event-data() -> ()  [unwired: 1 in, 6 out]
                  n273 = flat-sequence {
                    tunnel: w446 -> [w455]
                    tunnel: [w455] -> w445
                    tunnel: [w452] -> w444
                    tunnel: [w457] -> w448
                    tunnel: w445 -> [w458]
                    tunnel: w444 -> [w456]
                    tunnel: w448 -> [w477]
                    tunnel: [w477] -> w447
                    frame #0 {
                      n274 = call "EnterPassword.vi"("Message"="Press OK to Enter Password to save Prod Test paths \nor Cancel to Quit ", "Enable(t)"=TRUE) -> ("success(t)"=w450:bool, "cancelled(t)"=w453:bool)  [unwired: 7 in, 1 out]
                      n275 = Not(x=w453) -> (.not. x?=w451:bool)
                      n276 = And(x=w451, y=w450) -> (x .and. y?=w452:bool)
                    }
                    frame #1 {
                      n277 = case shown="True" w456 {
                        tunnel: w458 -> [w459 w462]
                        tunnel: [w459 w461] -> w457
                        frame False {
                        }
                        frame True {
                          n278 = control-ref of="Tests Path_Prod"() -> (w460:refnum<vi>)
                          n279 = local read "ctrl file path"() -> (w464:path)
                          n280 = Build Array(w460) -> (w465:refnum<vi>[])
                          n281 = disable-structure shown="Enabled" {
                            disable-tunnel: w465 -> [w470 w476]
                            disable-tunnel: w464 -> [w469 w471]
                            disable-tunnel: TRUE ("Use vi Path") -> [w468 w472]
                            disable-tunnel: w462 -> [w467 w474]
                            disable-tunnel: [w466 w473] -> w461
                            frame Disabled {
                              n282 = call "Load and Save Controls.vi"("path"=w469, "Use vi Path"=w468, "error in (no error)"=w467, "Control References"=w470) -> ("error out"=w466:errorcluster)  [unwired: 7 in]
                            }
                            frame Enabled {
                              n283 = call "Read and Write Controls to Automatic Config File.vi"("path"=w471, "Use Path"=w472, "Action"=RWC_Actions."Write", "error in"=w474, "Control References"=w476) -> ("error out"=w473:errorcluster)  [unwired: 5 in, 1 out]
                            }
                          }
                        }
                      }
                    }
                    frame #2 {
                      n284 = local write "cancelled(t)"(TRUE ("cancelled(t)")) -> ()
                      n285 = local write "Save Prod Tests"(FALSE ("Launch Switch GUI")) -> ()
                    }
                  }
                }
                event "Launch Post Processer GUI": Value Change {
                  n286 = event-data() -> ()  [unwired: 1 in, 6 out]
                  n287 = flat-sequence {
                    tunnel: [w481] -> w480
                    tunnel: w480 -> [w482]
                    frame #0 {
                    }
                    frame #1 {
                      n288 = call "FinalReportResult_GUI.vi"() -> ("This VI"=w481:refnum<vi>)  [unwired: 11 in, 4 out]
                    }
                    frame #2 {
                      n289 = invoke class="VI" method="Abort VI"(reference=w482) -> ()  [unwired: 2 in, 3 out]
                      n290 = local write "Launch Post Processer GUI"(FALSE ("Launch Switch GUI")) -> ()
                      n291 = local write "cancelled(t)"(TRUE ("cancelled(t)")) -> ()
                    }
                  }
                }
                event "Launch Tetra Lab GUI": Value Change {
                  n292 = event-data() -> ()  [unwired: 1 in, 6 out]
                  n293 = flat-sequence {
                    frame #0 {
                    }
                    frame #1 {
                      (unwired) path "C:/TetraLabGUI" ("working directory")
                      n294 = global read "Sequence Globals.vi" "AppSupportPath 3"() -> (w487:path)
                      n295 = global read "Sequence Globals.vi" "DevSupportPath"() -> (w491:path)
                      n296 = local read "IsRuntime?"() -> (w488:bool)
                      n297 = Build Path(base path=w491, name or relative path="TetraLabGUI") -> (appended path=w489:path)
                      n298 = Select(t=w487, s=w488, f=w489) -> (s? t:f=w486:path)
                      n299 = call <vilib>:"System Exec.vi"("run minimized? (F)"=FALSE, "wait until completion? (T)"=FALSE, "working directory"=w486, "command line"="python TetraLabGUI.py ") -> ()  [unwired: 4 in, 4 out]
                    }
                    frame #2 {
                      n300 = local write "cancelled(t)"(TRUE ("cancelled(t)")) -> ()
                    }
                  }
                }
                event "LaunchFieldTestApp": Value Change {
                  n301 = event-data() -> ()  [unwired: 1 in, 6 out]
                  n302 = flat-sequence {
                    frame #0 {
                      n303 = call "Display Message to User12"() -> ("OK"=w496:bool)  [unwired: 10 in, 1 out]
                      n304 = local write "cancelled(t)"(w496) -> ()
                    }
                    frame #1 {
                      n305 = global read "Sequence Globals.vi" "AppSupportPath 3"() -> (w503:path)
                      n306 = global read "Sequence Globals.vi" "DevSupportPath"() -> (w501:path)
                      n307 = local read "IsRuntime?"() -> (w504:bool)
                      n308 = Build Path(base path=w501, name or relative path="FieldTestApp") -> (appended path=w505:path)
                      n309 = Select(t=w503, s=w504, f=w505) -> (s? t:f=w500:path)
                      n310 = Path To String(path=w500) -> (string=w498:string)
                      n311 = Concatenate Strings(w498, "/FieldTest.exe" ("command line")) -> (w499:string)
                      n312 = call <vilib>:"System Exec.vi"("expected output size  (4096)"=u32 4096, "wait until completion? (T)"=FALSE, "command line"=w499) -> ()  [unwired: 5 in, 4 out]
                    }
                    frame #2 {
                      n313 = local write "LaunchFieldTestApp"(FALSE ("LaunchFieldTestApp")) -> ()
                    }
                  }
                }
              }
              "-ssid" <- w274
              "current time" <- w269
              n314 = global write "Tetra_Globals.vi" "-ssid"(w274) -> ()
              n315 = Get Date/Time String(seconds (now)=w269) -> (date string=w270:string, time string=w271:string)  [unwired: 2 in]
              n316 = call <vilib>:"Space Constant.vi"() -> ("String"=w272:string)
              n317 = Concatenate Strings(w270, w272, w271) -> (w273:string)
              "Seq Start Time" <- w273
              n318 = global write "Test Parameter Globals_1.0.0.vi" "Seq Start Time"(w273) -> ()
            }
            frame #2 {
              # "Run Cal Module IF:\nnot cancelled AND\nForce OR Enable Cal\nAND IF\nIs Production AND IF\nTx is Being Tested"
              n319 = local read "cancelled(t)"() -> (w523:bool)
              n320 = local read "Enable S11 Cal(t)"() -> (w512:bool)
              n321 = local read "Run All Tests (T)"() -> (w519:bool)
              n322 = local read "Run WAM TX (T)"() -> (w518:bool)
              n323 = local read "Prod_Mode(T)"() -> (w516:bool)
              n324 = local read "FirstCall(t)"() -> (w514:bool)
              n325 = local read "Force an S11 Cal(T)"() -> (w509:bool)
              n326 = Or(x=w519, y=w518) -> (x .or. y?=w517:bool)
              n327 = Not(x=w523) -> (.not. x?=w521:bool)
              n328 = global write "Tetra_Globals.vi" "Use Serial log(T)"("Use Serial log(T)") -> ()
              n329 = And(x=w517, y=w516) -> (x .and. y?=w515:bool)
              n330 = And(x=w521, y=w512) -> (x .and. y?=w522:bool)
              n331 = And(x=w515, y=w514) -> (x .and. y?=w513:bool)
              n332 = And(x=w522, y=w513) -> (x .and. y?=w510:bool)
              n333 = Or(x=w510, y=w509) -> (x .or. y?=w511:bool)
            }
          }
          n334 = Greater Than 0?(x=w253) -> (x > 0?=w251:bool)
          n335 = case shown="False" w250 {
            tunnel: [w526 w532] -> w256
            tunnel: [TRUE ("Success?(t)") w531] -> w254
            tunnel: w252 -> [w526 w530]
            tunnel: w251 -> [_ w529]
            frame False {
            }
            frame True {
              n336 = flat-sequence "Calibration" {
                tunnel: [w542] -> w534
                tunnel: [w540] -> w533
                tunnel: w530 -> [w537]
                tunnel: w529 -> [w541]
                tunnel: w534 -> [w595]
                tunnel: w533 -> [w598]
                tunnel: [w596] -> w532
                tunnel: [w597] -> w531
                tunnel: [w592] -> w527
                tunnel: [w591] -> w528
                frame #0 {
                  n337 = local read "Inst_vi"() -> (w535:path)
                  n338 = for {
                    N: 2 -> [_]
                    tunnel: [w545] -> w538
                    tunnel: w537 -> [w547]
                    tunnel: [w544] -> w536
                    tunnel: w535 -> [w543]
                    stop <- w545 stop-if-true
                    n339 = flat-sequence {
                      tunnel: w547 -> [w554]
                      tunnel: [w553] -> w546
                      tunnel: w543 -> [w552]
                      frame #0 {
                        n340 = global read "Station References Global.vi" "RF Switch Present?"() -> (w555:bool)
                        n341 = global read "Station References Global.vi" "PNA Present?"() -> (w556:bool)
                        n342 = And(x=w556, y=w555) -> (x .and. y?=w557:bool)
                        n343 = case shown="False" w557 {
                          tunnel: w554 -> [w562 w563]
                          tunnel: [w561 w563] -> w553
                          tunnel: w552 -> [w560 _]
                          frame False {
                            w559 = TRUE  # Auto Dispose Reference
                            n344 = call "Open vi Reference_3.0.0.0.vi"("Close Front Panel(T)"=TRUE, "Wait Until Done"=w559, "Auto Dispose Reference"=w559, "error in"=w562, "vi path"=w560) -> ("error out"=w561:errorcluster)  [unwired: 4 in, 2 out]
                          }
                          frame True {
                          }
                        }
                      }
                    }
                    n345 = flat-sequence {
                      tunnel: [w548] -> _
                      tunnel: w546 -> [w548]
                      tunnel: [w549] -> w545
                      tunnel: [w548] -> w544
                      frame #0 {
                        n346 = global read "Station References Global.vi" "RF Switch Present?"() -> (w551:bool)
                        n347 = global read "Station References Global.vi" "PNA Present?"() -> (w550:bool)
                        n348 = And(x=w550, y=w551) -> (x .and. y?=w549:bool)
                      }
                    }
                  }
                  n349 = case shown="True" w538 {
                    tunnel: [FALSE ("Cal_Flag(t)") w589] -> w542
                    tunnel: w536 -> [w565 w585]
                    tunnel: w541 -> [_ w581]
                    tunnel: [w565 w575] -> w540
                    frame False {
                    }
                    frame True {
                      w590 = TRUE ("RunCalCheck(t)")
                      # "need visa adress if instruments globals has not run"
                      n350 = Select(t="Re- Running Cal..." ("Text.Text"), s=w581, f="Checking Cal..." ("Text.Text")) -> (s? t:f=w573:string)
                      n351 = global read "Station References Global.vi" "RF Switch"() -> (w566:refnum<visa-resource-name>)
                      n352 = global read "Station References Global.vi" "PNA"() -> (w567:refnum<visa-resource-name>)
                      n353 = control-ref of="Test Run 2"() -> (w583:refnum<vi>)
                      n354 = property class="Str"(reference=w583, error in=w585, "Text.Text"=w573) -> (reference out=w579:refnum<vi>, error out=w584:errorcluster)
                      n355 = call "PNA_CalFile_Check.vi"("PNA_IN"=w567, "RF_SW_IN"=w566, "error in"=w584, "HrsToFlag"="HrsToFlag", "PopUp Alert(t)"=FALSE, "RunFileCheck(t)"=w590, "RunCalCheck(t)"=w590, "DoCal(t)"=FALSE) -> ("File Date/Time"=w577:string, "Cal_Flag(t)"=w589:bool, "error out"=w576:errorcluster)  [unwired: 9 in]
                      n356 = Concatenate Strings(w573, "\r\n", "The Last Calibration was saved at    " ("string"), w577) -> (w569:string)
                      n357 = local read "Force an S11 Cal(T)"() -> (w571:bool)
                      n358 = Select(t="The Forced Calibration bit is checked" ("string"), s=w571, f=w569) -> (s? t:f=w570:string)
                      n359 = property class="Str"(reference=w579, error in=w576, "Text.Text"=w570) -> (error out=w574:errorcluster)  [unwired: 1 out]
                      n360 = call "Time Delay3"("error in (no error)"=w574) -> ("error out"=w575:errorcluster)  [unwired: 10 in]
                    }
                  }
                }
                frame #1 {
                  # "!! The s11 Calibration was Bypassed"
                  n361 = local read "Force an S11 Cal(T)"() -> (w593:bool)
                  n362 = Or(x=w595, y=w593) -> (x .or. y?=w594:bool)
                  n363 = case shown="True" w594 {
                    tunnel: w598 -> [w601 w610]
                    tunnel: [TRUE ("Success?(t)") w603] -> w597
                    tunnel: [w601 w608] -> w596
                    tunnel: w593 -> [_ w606]
                    tunnel: ["" w605] -> w592
                    tunnel: [FALSE ("Enable") w604] -> w591
                    frame False {
                    }
                    frame True {
                      n364 = case shown="False" w606 {
                        selector: w606 -> [_ w615]
                        tunnel: w610 -> [w613 w614]
                        tunnel: [w612 w614] -> w609
                        tunnel: [w611 w615] -> w607
                        frame False {
                          n365 = call "Display Message to User10"("error in (no error)"=w613) -> ("error out"=w612:errorcluster, "OK"=w611:bool)  [unwired: 9 in]
                        }
                        frame True {
                        }
                      }
                      n366 = case shown="True" w607 {
                        tunnel: [w626 w635] -> w608
                        tunnel: w609 -> [w628 w639]
                        tunnel: [w618 w636] -> w605
                        tunnel: [TRUE ("S11_Success(t)") w631] -> w604
                        tunnel: [w616 w631] -> w603
                        frame False {
                          n367 = call "EnterPassword.vi"("error in (no error)"=w628, "Enable(t)"=TRUE) -> ("error out"=w626:errorcluster, "success(t)"=w616:bool, "cancelled(t)"=w621:bool)  [unwired: 7 in]
                          n368 = local write "cancelled(t)"(w621) -> ()
                          n369 = Select(t="S11 Cal Bypass Successful" ("Text.Text"), s=w616, f="S11 Bypass Cal Unsuccessful" ("Text.Text")) -> (s? t:f=w625:string)
                          n370 = control-ref of="Test Run 2"() -> (w624:refnum<vi>)
                          n371 = Select(t="Connect a WAM module to begin." ("Text.Text"), s=w616, f="Cancelled or Incorrect password. Try Again" ("Text.Text")) -> (s? t:f=w618:string)
                          n372 = property class="Str"(reference=w624, "Text.Text"=w625) -> ()  [unwired: 1 in, 2 out]
                        }
                        frame True {
                          n373 = while {
                            tunnel: w639 -> [w647]
                            tunnel: [w645] -> w635
                            tunnel: [w640] -> w631
                            i -> [w644]
                            stop <- w642 stop-if-true
                            w646 = TRUE ("Enable(t)")
                            n374 = call "CalPoPup.vi"("error in (no error)"=w647, "Enable(t)"=w646, "RunCALvi(t)"=w646) -> ("Success?(t)"=w641:bool, "error out"=w645:errorcluster)  [unwired: 15 in]
                            n375 = case shown="True" w641 {
                              tunnel: [w653 w656] -> w643
                              tunnel: w641 -> [_ w656]
                              frame False {
                                n376 = call "Display Message to User15"("Enable"=TRUE, "Message"="There was a problem with the Calibration.\nPress OK to Cancel or Repeat Cal to Repeat") -> ("OK"=w653:bool)  [unwired: 8 in, 1 out]
                                n377 = local write "cancelled(t)"(w653) -> ()
                              }
                              frame True {
                                n378 = call "Display Message to User14"("Enable"=TRUE, "Message"="Cal Successful! Press OK to Continue or Repeat Cal to Repeat") -> ()  [unwired: 8 in, 2 out]
                                "S11_Success(t)" <- w656
                              }
                            }
                            n379 = case shown="2" w644 {
                              tunnel: [w648 w651] -> w642
                              tunnel: w643 -> [w648 _]
                              tunnel: [w648 w649] -> w640
                              frame 0, Default {
                                n380 = local write "S11_Success(t)"(w648) -> ()
                              }
                              frame 2 {
                                n381 = call "Display Message to User16"("Enable"=TRUE, "Message"="Max 3 times to try calibration.\nStart the sequence Over!") -> ("OK"=w651:bool)  [unwired: 8 in, 1 out]
                                n382 = Not(x=w651) -> (.not. x?=w649:bool)
                                n383 = local write "cancelled(t)"(w651) -> ()
                                n384 = local write "S11_Success(t)"(w649) -> ()
                              }
                            }
                          }
                          n385 = Not(x=w631) -> (.not. x?=w632:bool)
                          n386 = Select(t="S11 Cal Successful" ("Text.Text"), s=w631, f="S11 Cal Not Successful" ("Text.Text")) -> (s? t:f=w634:string)
                          n387 = local write "Force an S11 Cal(T)"(w632) -> ()
                          n388 = control-ref of="Test Run 2"() -> (w633:refnum<vi>)
                          n389 = property class="Str"(reference=w633, "Text.Text"=w634) -> ()  [unwired: 1 in, 2 out]
                          n390 = Select(t="Connect the WAM Module for Test and Press Continue", s=w631, f="The Cal was Not Successful") -> (s? t:f=w636:string)
                        }
                      }
                    }
                  }
                }
              }
              n391 = call "Display Message to User11"("Enable"=w528, "Message"=w527) -> ()  [unwired: 8 in, 2 out]
            }
          }
        }
        n392 = global write "Tetra_Globals.vi" "Ser log Folder"("Ser log Folder") -> ()
      }
      frame #5 {
      }
      frame #6 {
        n393 = local read "cancelled(t)"() -> (w660:bool)
        n394 = case shown="False" w660 {
          tunnel: w664 -> [w704 w813]
          tunnel: [w697 _] -> w663
          tunnel: [w683 w813] -> w662
          tunnel: [w695 TRUE] -> w661
          frame False {
            w670 = "C" ("true string")
            n395 = stacked-sequence {
              tunnel: [w712] -> w674
              frame #0 {
                (unwired) path "C:/RageATE/Automated Tests/Tetra WAM/Utilities/BarCode.txt" ("Test Parameters File")
                n396 = global read "Sequence Globals.vi" "DevSupportPath"() -> (w710:path)
                n397 = local read "IsRuntime?"() -> (w711:bool)
                n398 = global read "Sequence Globals.vi" "AppSupportPath"() -> (w714:path)
                n399 = Strip Path(path=w710) -> (stripped path=w709:path)  [unwired: 1 out]
                n400 = Build Path(base path=w709, name or relative path="Automated Tests\\Tetra WAM\\Utilities\\BarCode.txt") -> (appended path=w707:path)
                n401 = Strip Path(path=w707) -> (name=w715:string)  [unwired: 1 out]
                n402 = Build Path(base path=w714, name or relative path=w715) -> (appended path=w713:path)
                n403 = Select(t=w713, s=w711, f=w707) -> (s? t:f=w712:path)
              }
            }
            n404 = Empty String/Path?(string/path="Build rev suffix") -> (empty?=w692:bool)
            n405 = case shown="False" w692 {
              tunnel: "Build rev suffix" -> [w717 w725]
              tunnel: [w721 w725] -> w690
              frame False {
                n406 = Concatenate Strings("You Have Chosen to use a suffix of " ("string"), w717, " On the Build revision code.\nPress OK to continue or CLEAR to Erase the suffix" ("string")) -> (w718:string)
                n407 = Two Button Dialog(message=w718, 1:"CLEAR" ("F button name (\"Cancel\")")) -> (T button?=w722:bool)  [unwired: 1 in]
                n408 = case shown="True" w722 {
                  tunnel: w717 -> [_ w724]
                  tunnel: ["" w724] -> w721
                  frame False {
                  }
                  frame True {
                  }
                }
              }
              frame True {
              }
            }
            n409 = local read "WAM_Bar_Code_Read"() -> (w700:bool)
            n410 = local read "User Prompt for SN (T)"() -> (w699:bool)
            n411 = local read "START TESTING"() -> (w705:bool)
            n412 = case shown="True" w699 {
              selector: w699 -> [w735 w751]
              tunnel: [_ w752] -> w706
              tunnel: w700 -> [_ w750]
              tunnel: w704 -> [w734 w749]
              tunnel: [w734 w748] -> w689
              tunnel: [_ w747] -> w697
              tunnel: w705 -> [_ w742]
              tunnel: [_ w746] -> w703
              tunnel: [_ w745] -> w702
              tunnel: [_ w744] -> w694
              tunnel: [_ w743] -> w698
              tunnel: w690 -> [_ w741]
              tunnel: [w731 w740] -> w679
              tunnel: w674 -> [w732 w739]
              tunnel: [FALSE w738] -> w677
              tunnel: [w732 w737] -> w675
              tunnel: [w731 w736] -> w665
              frame False {
                w731 = FALSE ("cancelled?(t)")
                n413 = global write "Test Parameter Globals_1.0.0.vi" "User Prompt for SN (T)"(w735) -> ()
              }
              frame True {
                n414 = case shown="True" w742 {
                  tunnel: [w766 w786] -> w752
                  tunnel: w751 -> [_ w785]
                  tunnel: w750 -> [_ w784]
                  tunnel: w749 -> [w765 w783]
                  tunnel: [w765 w782] -> w748
                  tunnel: [w756 w781] -> w747
                  tunnel: [w764 w780] -> w746
                  tunnel: [w763 w779] -> w745
                  tunnel: [w762 w778] -> w744
                  tunnel: [w761 w777] -> w743
                  tunnel: w741 -> [_ w776]
                  tunnel: [FALSE ("cancelled?(t)") w775] -> w740
                  tunnel: w739 -> [w759 w773]
                  tunnel: [TRUE w774] -> w738
                  tunnel: [w754 w773] -> w737
                  tunnel: [w753 w772] -> w736
                  frame False {
                    n415 = call <vilib>:"Check if File or Folder Exists.vi"("path"=w759) -> ("file or folder exists?"=w758:bool, "dup path"=w757:path)  [unwired: 8 in, 1 out]
                    n416 = case shown="True" w758 {
                      tunnel: w757 -> [w769 w770]
                      tunnel: [_ w771] -> w756
                      tunnel: [w769 w770] -> w754
                      frame False {
                        w768 = T10."open or create"  # operation (0:open)
                        n417 = Open/Create/Replace File(file path (use dialog)=w769, operation (0:open)=w768) -> (refnum out=w767:refnum<file>)  [unwired: 4 in, 2 out]
                        n418 = Close File(refnum=w767) -> ()  [unwired: 1 in, 2 out]
                      }
                      frame True {
                        n419 = Read from Text File(file (use dialog)=w770) -> (text=w771:string)  [unwired: 3 in, 3 out]
                      }
                    }
                    n420 = global read "Tetra_Globals.vi" "RevC(t)"() -> (w753:bool)
                    n421 = global read "Tetra_Globals.vi" "BarCodeESN"() -> (w761:string)
                    n422 = local read "BarCodeInfo"() -> (w762:string)
                    n423 = global read "Test Parameter Globals_1.0.0.vi" "Global SN"() -> (w766:string)
                    n424 = global read "Tetra_Globals.vi" "Revision"() -> (w763:string)
                    n425 = global read "Test Parameter Globals_1.0.0.vi" "LOT ID"() -> (w764:string)
                  }
                  frame True {
                    n426 = case shown="True" w784 {
                      selector: w784 -> [_ w811]
                      tunnel: [w796 w812] -> w786
                      tunnel: w785 -> [w797 _]
                      tunnel: w783 -> [w798 w810]
                      tunnel: [w799 w809] -> w782
                      tunnel: [w793 w806] -> w781
                      tunnel: [w795 w808] -> w780
                      tunnel: [w794 w807] -> w779
                      tunnel: [w792 w805] -> w778
                      tunnel: [w791 w804] -> w777
                      tunnel: w776 -> [w790 w803]
                      tunnel: [w789 w802] -> w775
                      tunnel: [w788 w801] -> w774
                      tunnel: [w787 w800] -> w772
                      frame False {
                        n427 = call "WAM_SN_Prompt.vi"("Enable"=w797, "error in (no error)"=w798, "Rev_suffix"=w790) -> ("Bar Code"=w793:string, "BarCodeInfo"=w792:string, "BC_MSN"=w796:string, "cancelled?(t)"=w789:bool, "LotID"=w795:string, "rev_c?(t)"=w787:bool, "BC_ESN"=w791:string, "Revision"=w794:string, "error out"=w799:errorcluster)  [unwired: 4 in]
                        n428 = Not(x=w789) -> (.not. x?=w788:bool)
                        n429 = local write "ABORT AT SN SCAN(T)"(w789) -> ()
                      }
                      frame True {
                        n430 = call "WAM_BarCode_Prompt.vi"("Enable"=w811, "error in (no error)"=w810, "Rev_suffix"=w803) -> ("Bar Code"=w806:string, "BarCodeInfo"=w805:string, "BC_MSN"=w812:string, "cancelled?(t)"=w802:bool, "LotID"=w808:string, "rev_c?(t)"=w800:bool, "BC_ESN"=w804:string, "Revision"=w807:string, "error out"=w809:errorcluster)  [unwired: 4 in]
                        n431 = Not(x=w802) -> (.not. x?=w801:bool)
                        n432 = local write "ABORT AT SN SCAN(T)"(w802) -> ()
                      }
                    }
                  }
                }
                n433 = global write "Test Parameter Globals_1.0.0.vi" "User Prompt for SN (T)"(w751) -> ()
              }
            }
            "BarCodeInfo" <- w694
            n434 = local write "Build rev suffix"(w690) -> ()
            n435 = call <vilib>:"Check if File or Folder Exists.vi"("error in (no error)"=w689, "path"=w675) -> ("error out"=w688:errorcluster, "file or folder exists?"=w696:bool, "dup path"=w676:path)  [unwired: 7 in]
            n436 = global write "Tetra_Globals.vi" "BarCodeESN"(w698) -> ()
            n437 = Not(x=w679) -> (.not. x?=w680:bool)
            n438 = global write "Test Parameter Globals_1.0.0.vi" "BarCodeInfo"(w694) -> ()
            n439 = global write "Test Parameter Globals_1.0.0.vi" "Global SN"(w706) -> ()
            n440 = Concatenate Strings(w702, w690) -> (w693:string)
            n441 = global write "Test Parameter Globals_1.0.0.vi" "LOT ID"(w703) -> ()
            n442 = call <vilib>:"Trim Whitespace.vi"("string"=w693) -> ("trimmed string"=w672:string)  [unwired: 1 in]
            n443 = And(x=w677, y=w696) -> (x .and. y?=w678:bool)
            n444 = case shown="True" w678 {
              tunnel: w676 -> [_ w730]
              tunnel: w697 -> [_ w729]
              tunnel: [w726 w728] -> w684
              tunnel: w688 -> [w726 w727]
              frame False {
              }
              frame True {
                n445 = Write to Text File(file (use dialog)=w730, text=w729, error in=w727) -> (error out=w728:errorcluster)  [unwired: 1 in, 2 out]
              }
            }
            n446 = Match Pattern(string=w672, regular expression="[.]") -> (before substring=w671:string)  [unwired: 1 in, 3 out]
            n447 = global write "Tetra_Globals.vi" "Revision"(w672) -> ()
            n448 = To Upper Case(1:w671) -> (0:w701:string)
            n449 = And(x=w680, y=TRUE ("Enable")) -> (x .and. y?=w682:bool)
            n450 = Match Pattern(string=w701, regular expression=w670) -> (match substring=w669:string)  [unwired: 1 in, 3 out]
            n451 = Equal?(x=w669, y=w670) -> ()  [unwired: 1 out]
            n452 = Select(t=FALSE, s="force_lc(t)", f=w665) -> (s? t:f=w668:bool)
            "REV-C?(T)" <- w668
            n453 = call "Three Button Dialog CORE-WithTimeout.vi"("message"="!!!PRESSING OK  WILL BEGIN THE TEST SEQUENCE!!!\n1. Make sure the WAM is connected and ready\n2. The Absorber panel is in place\n3. The Door to the Test Chamber are closed\n-IF Anything breaches the laight curtain after this point it        will trip the ESS (Electronic Safety System).\n-If the ESS is tripped you will be able to continue when prompted to reset it (time dependent) when the test payload starts (usually 30 seconds to 1 minute" ("Input Message"), "Timeout(s)"=10, "error in (no error)"=w684, "Enable(t)"=w682) -> ("OK(?)"=w685:bool, "error out"=w683:errorcluster)  [unwired: 9 in, 1 out]
            n454 = global write "Tetra_Globals.vi" "RevC(t)"(w668) -> ()
            n455 = Not(x=w685) -> (.not. x?=w695:bool)
          }
          frame True {
          }
        }
        n456 = local write "ABORT AT SN SCAN(T)"(w661) -> ()
      }
      frame #7 {
        n457 = local read "ABORT AT SN SCAN(T)"() -> (w815:bool)
        n458 = case shown="True" w815 {
          tunnel: w818 -> [w822 _]
          tunnel: w817 -> [w821 w858]
          tunnel: [w820 w858] -> w816
          frame False {
            n459 = local read "Use Admin Mode(T)"() -> (w819:bool)
            n460 = case shown="False" w819 {
              tunnel: w822 -> [w830 _]
              tunnel: w821 -> [w829 w857]
              tunnel: [w827 w857] -> w820
              frame False {
                n461 = call "Pre-FinalTestBcScan.vi"("error in (no error)"=w829, "WAM BarCode"=w830, "Enable(t)"=TRUE) -> ("Tested?(t)"=w823:bool, "STOP?(t)"=w825:bool, "Output String"=w826:string, "error out"=w828:errorcluster)  [unwired: 8 in, 1 out]
                n462 = case shown="False" w825 {
                  tunnel: w826 -> [w833 w856]
                  tunnel: w825 -> [_ w854]
                  tunnel: w828 -> [w834 w855]
                  tunnel: [w832 w851] -> w827
                  tunnel: w823 -> [w831 _]
                  frame False {
                    n463 = case shown="False" w831 {
                      tunnel: w834 -> [w837 w840]
                      tunnel: w833 -> [w836 w847]
                      tunnel: [w835 w841] -> w832
                      frame False {
                        n464 = local write "Test Run 2"(w836) -> ()
                        n465 = call "Time Delay4"("error in (no error)"=w837) -> ("error out"=w835:errorcluster)  [unwired: 10 in]
                      }
                      frame True {
                        n466 = local write "Test Run 2"(w847) -> ()
                        n467 = global read "Test Parameter Globals_1.0.0.vi" "Global SN"() -> (w845:string)
                        n468 = Concatenate Strings(w845, " Has Been Tested Before!" ("string"), "\r\n", "Press OK to Re-Test or Cancel to Start Over" ("string")) -> (w846:string)
                        n469 = call "Display Message to User9"("error in (no error)"=w840, "Message"=w846) -> ("error out"=w841:errorcluster, "OK"=w839:bool)  [unwired: 8 in]
                        n470 = Not(x=w839) -> (.not. x?=w838:bool)
                        n471 = local write "ABORT AT SN SCAN(T)"(w838) -> ()
                      }
                    }
                  }
                  frame True {
                    n472 = call "Display Message to User4"("error in (no error)"=w855, "Enable"=w854, "Message"=w856) -> ("error out"=w852:errorcluster, "END"=w848:bool)  [unwired: 7 in]
                    n473 = local write "ABORT AT SN SCAN(T)"(w848) -> ()
                    n474 = Not(x=w848) -> (.not. x?=w850:bool)
                    n475 = call "EnterPassword.vi"("error in (no error)"=w852, "Enable(t)"=w850) -> ("error out"=w851:errorcluster, "success(t)"=w853:bool)  [unwired: 7 in, 1 out]
                    n476 = Not(x=w853) -> (.not. x?=w849:bool)
                    n477 = local write "ABORT AT SN SCAN(T)"(w849) -> ()
                  }
                }
              }
              frame True {
              }
            }
          }
          frame True {
          }
        }
      }
      frame #8 {
        # "0) ATTEN\n1) BOUNCE\n2) TX-250\n3) RX-250\n4) TX-100\n5) RX-100"
        n478 = case shown="True" "Prod_Mode(T)" {
          tunnel: [w866 w878] -> w861
          tunnel: w864 -> [w867 w871]
          tunnel: [w867 w870] -> w863
          tunnel: [w865 w869] -> w860
          tunnel: [w865 w868] -> w859
          frame False {
            w865 = FALSE ("Run Final Test Result")
            n479 = local read "Test Count"() -> (w866:i32[])
          }
          frame True {
            # "250MHz (t) /100MHz (f)"
            n480 = local read "Test Resolution"() -> (w875:bool)
            n481 = case shown="False" "Run All Tests (T)" {
              selector: "Run All Tests (T)" -> [_ w922]
              tunnel: [w902 w930] -> w878
              tunnel: "Run WAM BOUNCE (T)" -> [w900 w928]
              tunnel: w875 -> [w895 w925]
              tunnel: "Run WAM-C Atten (t)" -> [w901 w929]
              tunnel: "Run WAM TX (T)" -> [w884 w909]
              tunnel: "Run WAM RX (T)" -> [w888 w915]
              tunnel: w871 -> [w880 w907]
              tunnel: [w880 w907] -> w870
              tunnel: [w879 w906] -> w869
              tunnel: [w879 w906] -> w868
              frame False {
                w879 = FALSE
                n482 = Boolean To (0,1)(Boolean=w901) -> (0, 1=w904:i16)
                n483 = Boolean To (0,1)(Boolean=w900) -> (0, 1=w903:i16)
                n484 = And(x=w884, y=w895) -> (x .and. y?=w899:bool)
                n485 = And(x=w888, y=w895) -> (x .and. y?=w897:bool)
                n486 = Boolean To (0,1)(Boolean=w899) -> (0, 1=w883:i16)
                n487 = Not(x=w899) -> (.not. x?=w898:bool)
                n488 = Boolean To (0,1)(Boolean=w897) -> (0, 1=w890:i16)
                n489 = Not(x=w897) -> (.not. x?=w896:bool)
                n490 = Boolean To (0,1)(Boolean=w898) -> (0, 1=w886:i16)
                n491 = Boolean To (0,1)(Boolean=w896) -> (0, 1=w894:i16)
                n492 = Select(t=w883, s=w884, f=i16 0) -> (s? t:f=w882:i16)
                n493 = Select(t=w890, s=w888, f=i16 0) -> (s? t:f=w889:i16)
                n494 = Select(t=w886, s=w884, f=i16 0) -> (s? t:f=w885:i16)
                n495 = Select(t=w894, s=w888, f=i16 0) -> (s? t:f=w893:i16)
                n496 = Build Array(w904, w903, w882, w889, w885, w893) -> (w905:i16[])
                n497 = To Long Integer(number=w905) -> (32bit integer=w902:i32[])
              }
              frame True {
                w906 = TRUE
                n498 = local write "Run WAM-C Atten (t)"(w922) -> ()
                n499 = Boolean To (0,1)(Boolean=w928) -> (0, 1=w931:i16)
                n500 = And(x=w909, y=w925) -> (x .and. y?=w927:bool)
                n501 = And(x=w915, y=w925) -> (x .and. y?=w924:bool)
                n502 = local write "Run WAM BOUNCE (T)"(w922) -> ()
                n503 = local write "Run WAM TX (T)"(w922) -> ()
                n504 = local write "Run WAM RX (T)"(w922) -> ()
                n505 = Boolean To (0,1)(Boolean=w927) -> (0, 1=w911:i16)
                n506 = Not(x=w927) -> (.not. x?=w926:bool)
                n507 = Boolean To (0,1)(Boolean=w924) -> (0, 1=w918:i16)
                n508 = Not(x=w924) -> (.not. x?=w923:bool)
                n509 = Boolean To (0,1)(Boolean=w926) -> (0, 1=w914:i16)
                n510 = Boolean To (0,1)(Boolean=w923) -> (0, 1=w921:i16)
                n511 = Select(t=w911, s=w909, f=i16 0) -> (s? t:f=w910:i16)
                n512 = Select(t=w918, s=w915, f=i16 0) -> (s? t:f=w917:i16)
                n513 = Boolean To (0,1)(Boolean=w929) -> (0, 1=w932:i16)
                n514 = Select(t=w914, s=w909, f=i16 0) -> (s? t:f=w913:i16)
                n515 = Select(t=w921, s=w915, f=i16 0) -> (s? t:f=w920:i16)
                n516 = Build Array(w932, w931, w910, w917, w913, w920) -> (w933:i16[])
                n517 = To Long Integer(number=w933) -> (32bit integer=w930:i32[])
              }
            }
          }
        }
        n518 = global write "Tetra_Globals.vi" "Prod_Mode(T)"("Prod_Mode(T)") -> ()
        n519 = local write "Run Final Test Result"(w859) -> ()
        n520 = local write "Send to Synology Drive"(w860) -> ()
      }
      frame #9 {
        n521 = local read "ABORT AT SN SCAN(T)"() -> (w939:bool)
        n522 = control-ref of="Test Run"() -> (w938:refnum<vi>)
        n523 = case shown="False" w939 {
          tunnel: w935 -> [w957 w1030]
          tunnel: [w956 w1030] -> w940
          tunnel: w934 -> [w941 _]
          frame False {
            n524 = local read "Prod_Mode(T)"() -> (w942:bool)
            n525 = local read "Tests Path_Eng"() -> (w943:path[])
            n526 = local read "Tests Path_Prod"() -> (w944:path[])
            n527 = local read "AppSupportPath"() -> (w945:path)
            n528 = local read "IsRuntime?"() -> (w946:bool)
            n529 = for {
              tunnel: w941 -> [w984] mode=indexing
              shift-right: [w990] -> w958
              shift-left: path[] [] -> [w991]
              tunnel: w944 -> [w982] mode=indexing
              tunnel: [w988] -> w947 mode=indexing
              tunnel: w957 -> [w977]
              tunnel: [w987] -> w950
              tunnel: w946 -> [w983]
              tunnel: w945 -> [w980]
              tunnel: w943 -> [w972] mode=indexing
              tunnel: w942 -> [w973]
              i -> [w989]
              n530 = Equal To 0?(x=w984) -> (x = 0?=w986:bool)
              n531 = Strip Path(path=w982) -> (name=w981:string)  [unwired: 1 out]
              n532 = case shown="True" w986 {
                tunnel: [w992 1] -> w985
                tunnel: w984 -> [w992 _]
                frame False {
                }
                frame True {
                }
              }
              n533 = Build Path(base path=w980, name or relative path=w981) -> (appended path=w979:path)
              n534 = Select(t=w979, s=w983, f=w982) -> (s? t:f=w975:path)
              n535 = Select(t=w975, s=w973, f=w972) -> (s? t:f=w974:path)
              n536 = call <vilib>:"Check if File or Folder Exists.vi"("error in (no error)"=w977, "path"=w974) -> ("error out"=w976:errorcluster, "dup path"=w978:path)  [unwired: 7 in, 1 out]
              n537 = for {
                N: w985 -> [_]
                tunnel: w984 -> [w996]
                shift-right: [w1000] -> w990
                shift-left: w991 -> [w1001]
                tunnel: w989 -> [w999]
                tunnel: [w998] -> w988
                tunnel: w978 -> [w997]
                tunnel: w976 -> [w995]
                tunnel: [w994] -> w987
                n538 = case shown="1.." w996 {
                  selector: w996 -> [_ w1015]
                  tunnel: [w1006 w1024] -> w1000
                  tunnel: w1001 -> [w1006 w1025]
                  tunnel: w999 -> [w1009 w1022]
                  tunnel: [w1007 w1020] -> w998
                  tunnel: w997 -> [_ w1013]
                  tunnel: w995 -> [w1003 w1012]
                  tunnel: [w1003 w1012] -> w994
                  frame 0, Default {
                    n539 = Increment(x=w1009) -> (x+1=w1002:i32)
                    n540 = Number To Decimal String(number=w1002) -> (decimal integer string=w1008:string)  [unwired: 1 in]
                    n541 = Concatenate Strings("Skip" ("string"), "Test ", w1008, " will Not run !" ("string")) -> (w1007:string)
                  }
                  frame 1.. {
                    n542 = Increment(x=w1022) -> (x+1=w1011:i32)
                    n543 = Insert Into Array(array=w1025, new element=w1013) -> (w1024:path[])  [unwired: 1 in]
                    n544 = Number To Decimal String(number=w1011) -> (decimal integer string=w1021:string)  [unwired: 1 in]
                    n545 = Number To Decimal String(number=w1015) -> (decimal integer string=w1014:string)  [unwired: 1 in]
                    n546 = Strip Path(path=w1013) -> (name=w1018:string)  [unwired: 1 out]
                    n547 = Concatenate Strings("Test ", w1021, " , " ("string"), w1018, " will run " ("string"), w1014, " times" ("string")) -> (w1020:string)
                  }
                }
              }
            }
            "TestsArray" <- w958
            n548 = Array Size(array=w958) -> (size(s)=w953:i32)
            "size(s)" <- w953
            n549 = Equal To 0?(x=w953) -> (x = 0?=w954:bool)
            n550 = Greater?(x=w953, y=0) -> (0:w951:bool)
            "More than 1 test?(T)" <- w951
            n551 = case shown="True" w954 {
              tunnel: w950 -> [w1026 w1028]
              tunnel: [w1026 w1028] -> w949
              frame False {
              }
              frame True {
                n552 = One Button Dialog(message="You must select at least 1 test parameter spreadsheet") -> (true=w1027:bool)  [unwired: 1 in]
                n553 = local write "ABORT AT SN SCAN(T)"(w1027) -> ()
              }
            }
            n554 = local read "Prod_Mode(T)"() -> (w948:bool)
            n555 = case shown="True" w948 {
              tunnel: w951 -> [w970 _]
              tunnel: w949 -> [w959 w971]
              tunnel: [w959 w971] -> w956
              tunnel: w947 -> [w962 _]
              frame False {
                w968 = "\r\n"
                n556 = Array To Spreadsheet String(delimiter (Tab)="\r\n", array=w962, 3:"%s" ("format string")) -> (spreadsheet string=w969:string)
                n557 = Concatenate Strings(w969, w968, "Press OK to Continue" ("string"), w968, "OR END to Stop Testing" ("string")) -> (w965:string)
                n558 = call "Display Message to User"("Enable"=w970, "Message"=w965) -> ("END"=w961:bool)  [unwired: 8 in, 1 out]
                n559 = Not(x=w961) -> (.not. x?=w960:bool)
                n560 = local write "ABORT AT SN SCAN(T)"(w960) -> ()
              }
              frame True {
              }
            }
          }
          frame True {
          }
        }
        n561 = property class="Str"(reference=w938, "Text.Text"="Starting Sequencer...", "Text.TextColor"=u32 0) -> ()  [unwired: 1 in, 2 out]
      }
      frame #10 {
        n562 = local read "ABORT AT SN SCAN(T)"() -> (w1031:bool)
        n563 = case shown="False" w1031 {
          tunnel: [w1038 w1196] -> w1034
          tunnel: w1033 -> [w1037 w1196]
          tunnel: [w1036 _] -> w1032
          frame False {
            n564 = local read "TestsArray"() -> (w1035:path[])
            n565 = while {
              tunnel: w1035 -> [w1046] mode=indexing
              tunnel: [w1053] -> w1038
              tunnel: w1037 -> [w1048]
              tunnel: [w1040] -> w1036 mode=indexing
              i -> [w1054]
              stop <- w1057 stop-if-true
              n566 = global write "Test Parameter Globals_1.0.0.vi" "Test Parameters File"(w1046) -> ()
              n567 = local read "size(s)"() -> (w1044:i32)
              n568 = Add(x=1, y=w1054) -> (x+y=w1045:i32)
              n569 = Equal?(x=w1044, y=w1045) -> (x = y?=w1056:bool)
              n570 = local read "Stop Sequencer"() -> (w1043:bool)
              n571 = flat-sequence {
                tunnel: w1048 -> [w1069]
                tunnel: [w1068] -> w1047
                tunnel: w1046 -> [w1077]
                tunnel: w1045 -> [w1075]
                tunnel: [w1083] -> w1063
                tunnel: [w1080] -> w1062
                tunnel: [w1084] -> w1061
                tunnel: [w1082] -> w1060
                tunnel: [w1081] -> w1059
                tunnel: [w1087] -> w1050
                tunnel: w1047 -> [w1087]
                tunnel: [w1084] -> w1039
                tunnel: [w1097] -> w1049
                tunnel: w1039 -> [w1093]
                tunnel: w1050 -> [w1090]
                tunnel: w1059 -> [w1091]
                tunnel: w1060 -> [w1092]
                tunnel: w1061 -> [w1094]
                tunnel: w1062 -> [w1095]
                tunnel: w1063 -> [w1096]
                tunnel: [w1156] -> w1058
                tunnel: [w1157] -> w1052
                tunnel: w1049 -> [w1157]
                tunnel: w1058 -> [w1161]
                tunnel: w1052 -> [w1160]
                tunnel: [w1159] -> w1051
                tunnel: [w1170] -> w1042
                tunnel: w1051 -> [w1170]
                tunnel: w1042 -> [w1171]
                tunnel: [w1171] -> w1041
                tunnel: [w1183] -> w1053
                tunnel: w1041 -> [w1176]
                tunnel: [w1175] -> w1040
                frame #0 {
                  w1065 = u32 16860
                  n572 = control-ref of="Test Run 2"() -> (w1064:refnum<vi>)
                  n573 = control-ref of="Test Run"() -> (w1070:refnum<vi>)
                  n574 = local read "size(s)"() -> (w1071:i32)
                  n575 = property class="Str"(reference=w1070, error in=w1069, "Text.TextColor"=w1065) -> (error out=w1068:errorcluster)  [unwired: 1 out]
                  n576 = property class="Str"(reference=w1064, "Text.TextColor"=w1065) -> ()  [unwired: 1 in, 2 out]
                  n577 = Path To String(path=w1077) -> (string=w1078:string)
                  n578 = Number To Decimal String(number=w1075) -> (decimal integer string=w1074:string)  [unwired: 1 in]
                  n579 = Number To Decimal String(number=w1071) -> (decimal integer string=w1072:string)  [unwired: 1 in]
                  n580 = Concatenate Strings("Running Test: " ("string"), w1078, "   " ("string"), w1074, " of " ("string"), w1072) -> (→"Test Run" →"Test Run 2":string)
                }
                frame #1 {
                  n581 = local read "Vi Sequence"() -> (w1079:T2)
                  n582 = Unbundle By Name(w1079) -> ("Vis to run in sequence"=w1083:path[], "Run"=w1080:bool[], "Panel Behavior"=w1082:u16[], "Close Panel(T)"=w1081:bool[])
                  n583 = control-ref of="This VI"() -> (w1085:refnum<vi>)
                  n584 = property class="VI"(reference=w1085, "FP.State"=T5."Minimized" ("Front Panel Window:State")) -> ()  [unwired: 1 in, 2 out]
                  n585 = Array Size(array=w1083) -> (size(s)=w1084:i32)
                }
                frame #2 {
                  # "Run the vi's in sequence"
                  n586 = global read "Sequence Globals.vi" "Stop Testing"() -> (w1088:bool)
                  n587 = case shown="False" w1088 {
                    tunnel: [w1111 _] -> w1100
                    tunnel: [w1110 _] -> w1099
                    tunnel: w1096 -> [w1109 _]
                    tunnel: w1095 -> [w1108 _]
                    tunnel: w1094 -> [w1107 _]
                    tunnel: w1093 -> [w1106 _]
                    tunnel: w1092 -> [w1105 _]
                    tunnel: w1091 -> [w1104 _]
                    tunnel: w1090 -> [w1103 _]
                    tunnel: [w1102 _] -> w1089
                    frame False {
                      n588 = for {
                        N: w1106 -> [_]
                        tunnel: w1109 -> [w1121] mode=indexing
                        tunnel: w1108 -> [w1116] mode=indexing
                        tunnel: [w1115] -> w1111 mode=indexing
                        tunnel: [w1127] -> w1110 mode=indexing
                        tunnel: w1107 -> [w1130]
                        tunnel: w1105 -> [w1129] mode=indexing
                        tunnel: w1104 -> [w1128] mode=indexing
                        tunnel: w1103 -> [w1125]
                        tunnel: [w1117] -> w1102 mode=indexing
                        tunnel: [w1114] -> w1101 mode=indexing
                        i -> [w1133]
                        stop <- w1112 stop-if-true
                        n589 = global read "Sequence Globals.vi" "Stop Testing"() -> (w1112:bool)
                        "Stop Testing" <- w1112
                        n590 = local read "AppSupportPath"() -> (w1119:path)
                        n591 = Add(x=1, y=w1133) -> (x+y=w1131:i32)
                        n592 = Equal?(x=w1130, y=w1131) -> ()  [unwired: 1 out]
                        n593 = Strip Path(path=w1121) -> (name=w1120:string)  [unwired: 1 out]
                        n594 = local read "IsRuntime?"() -> (w1122:bool)
                        n595 = Build Path(base path=w1119, name or relative path=w1120) -> (appended path=w1118:path)
                        n596 = Select(t=w1118, s=w1122, f=w1121) -> (s? t:f=w1114:path)
                        n597 = Not A Number/Path/Refnum?(number/path/refnum=w1114) -> (NaN/Path/Refnum?=w1124:bool)
                        n598 = Not(x=w1124) -> (.not. x?=w1123:bool)
                        n599 = And(x=w1116, y=w1123) -> (x .and. y?=w1113:bool)
                        n600 = case shown="True" w1113 {
                          tunnel: w1114 -> [_ w1143]
                          tunnel: [_ w1138] -> w1115
                          tunnel: [errorcluster {"status"=FALSE, "code"=0, "source"=""} ("error out") w1136] -> w1127
                          tunnel: w1129 -> [_ w1142]
                          tunnel: w1128 -> [_ w1135]
                          tunnel: w1125 -> [_ w1139]
                          frame False {
                          }
                          frame True {
                            n601 = call "Open vi Reference_2.2.0.0.vi"("Close Front Panel(T)"=w1135, "Wait Until Done"=TRUE, "Front Panel State"=w1142, "Auto Dispose Reference"=FALSE, "error in"=w1139, "vi path"=w1143) -> ("error out"=w1137:errorcluster, "vi reference"=w1138:refnum<vi>)  [unwired: 2 in, 2 out]
                            n602 = case shown="True" w1135 {
                              tunnel: w1138 -> [_ w1146]
                              tunnel: w1137 -> [w1144 w1145]
                              tunnel: [w1144 w1145] -> w1136
                              frame False {
                              }
                              frame True {
                                n603 = invoke class="VI" method="FP.Close"(reference=w1146) -> ()  [unwired: 2 in, 3 out]
                              }
                            }
                          }
                        }
                        n604 = Unbundle By Name(w1127) -> ("status"=w1126:bool)
                        n605 = Or(x=w1112, y=w1126) -> ()  [unwired: 1 out]
                        n606 = Path To String(path=w1114) -> (string=w1117:string)
                        "run?" <- w1116
                      }
                      "vis to run" <- w1101
                    }
                    frame True {
                    }
                  }
                  "viRefs" <- w1100
                  "Array" <- w1089
                  n607 = for {
                    tunnel: [w1149] -> w1098 mode=indexing
                    tunnel: w1100 -> [w1148] mode=indexing
                    tunnel: w1099 -> [w1150] mode=indexing
                    tunnel: [w1149] -> w1097
                    n608 = Not A Number/Path/Refnum?(number/path/refnum=w1148) -> (NaN/Path/Refnum?=w1147:bool)
                    n609 = case shown="False" w1147 {
                      tunnel: w1150 -> [w1153 w1154]
                      tunnel: [w1152 w1154] -> w1149
                      tunnel: w1148 -> [w1151 _]
                      frame False {
                        n610 = Close Reference(reference=w1151, error in (no error)=w1153) -> (error out=w1152:errorcluster)
                      }
                      frame True {
                      }
                    }
                  }
                  "Close errors" <- w1098
                }
                frame #3 {
                  n611 = global read "Test Result File Name Global.vi" "Test Results File Name"() -> (w1156:path)
                  "Test Results File Name (Local computer,Automatically generated)" <- w1156
                  n612 = Path To String(path=w1156) -> (string=→"TestResultLink":string)
                }
                frame #4 {
                  # "C:\\Users\\ThomasWattson\\Rage Systems\\Rage Test Lab - Documents\\ATE Results"
                  n613 = case shown="True" "PLace a result file\n copy on server(T)" {
                    tunnel: w1161 -> [w1163 w1166]
                    tunnel: [w1164 w1169] -> w1159
                    tunnel: w1160 -> [w1164 w1168]
                    tunnel: [w1163 w1165] -> w1158
                    frame False {
                    }
                    frame True {
                      w1167 = path "C:/Users/ThomasWattson/TomWOneDrive/OneDrive - Rage Systems/Documents - Tetra/Test Docs/Test Results/WAM/ATE Results Backup"  # Result Archive location
                      n614 = call "ArchiveResults.vi"("error in"=w1168, "Archive Path"=w1167, "source path"=w1166) -> ("error out"=w1169:errorcluster, "Archive PathOut"=w1165:path)  [unwired: 6 in, 1 out]
                    }
                  }
                  "Results Archive File (Location on server)" <- w1158
                }
                frame #5 {
                }
                frame #6 {
                }
                frame #7 {
                  w1179 = ".tst"  # replace string ("")
                  w1180 = ".csv"  # name or relative path
                  n615 = local read "Test Results File Name (Local computer,Automatically generated)"() -> (w1175:path)
                  n616 = case shown="True" "Generate a log file entry for this test" {
                    tunnel: [path "" ("logfileout") w1191] -> w1173
                    frame False {
                    }
                    frame True {
                      n617 = local read "LogFilePath"() -> (w1190:path)
                      n618 = call "Write Test Log.vi"("file path (dialog if empty)"=w1190) -> ("logfileout"=w1191:path)  [unwired: 10 in]
                    }
                  }
                  n619 = global read "Test Parameter Globals_1.0.0.vi" "Test Parameters File"() -> (w1182:path)
                  n620 = case shown="False" "Open output file\n when test done" {
                    tunnel: [w1192 w1195] -> w1184
                    tunnel: w1176 -> [w1192 w1194]
                    tunnel: w1175 -> [_ w1193]
                    frame False {
                    }
                    frame True {
                      n621 = call "Open_Results_File_Excel.vi"("error in (no error)"=w1194, "path to file"=w1193) -> ("error out"=w1195:errorcluster)  [unwired: 9 in]
                    }
                  }
                  n622 = Path To String(path=w1175) -> (string=w1181:string)
                  n623 = Search and Replace String(input string=w1181, search string=w1180, replace string=w1179) -> (result string=w1178:string)  [unwired: 5 in, 3 out]
                  n624 = Path To String(path=w1173) -> (string=→"logfileout":string)
                  n625 = String To Path(string=w1178) -> (path=w1177:path)
                  n626 = call-poly <vilib>:"Read Delimited Spreadsheet.vi"("file path (dialog if empty)"=w1182, "error in (no error)"=w1176) -> ("all rows"=w1187:string[][], "error out"=w1186:errorcluster)  [unwired: 8 in, 4 out]
                  n627 = call-poly <vilib>:"Write Delimited Spreadsheet.vi"("file path (dialog if empty)"=w1177, "2D data"=w1187, "error in (no error)"=w1186) -> ("error out"=w1185:errorcluster)  [unwired: 11 in, 1 out]
                  n628 = Merge Errors(w1184, w1185) -> (w1183:errorcluster)
                }
              }
              n629 = Or(x=w1056, y=w1043) -> (x .or. y?=w1057:bool)
            }
          }
          frame True {
          }
        }
        "result files array" <- w1032
      }
      frame #11 {
        n630 = local read "ABORT AT SN SCAN(T)"() -> (w1197:bool)
        n631 = case shown="False" w1197 {
          tunnel: [w1221 w1234] -> w1199
          tunnel: w1198 -> [w1205 w1234]
          frame False {
            w1208 = u32 4 items=["OFF"=0, "RED"=1, "AMBER"=2, "GREEN"=4, "GRE+AMBER"=6, "ALL"=7, "BUZZ"=8, "RED+BUZZ"=9, "ALL+BUZZ"=15] ("Select")
            w1215 = u32 0
            n632 = global read "Tetra_Globals.vi" "comport"() -> (w1201:refnum<visa-resource-name>)
            n633 = disable-structure shown="Enabled" {
              frame Disabled {
                n634 = call "Display Message to User2"() -> ()  [unwired: 10 in, 2 out]
              }
              frame Enabled {
              }
            }
            n635 = local read "Array Element.Value"() -> (w1206:variant)
            n636 = Wait (ms)(milliseconds to wait=u32 2000) -> ()  [unwired: 1 out]
            n637 = global read "Station References Global.vi" "Gantry"() -> (w1202:refnum<visa-resource-name>)
            n638 = VISA Close(VISA resource name=w1201) -> ()  [unwired: 1 in, 1 out]
            n639 = control-ref of="Run"() -> (w1207:refnum<vi>)
            n640 = case shown="False" "SendGantryHome(t)" {
              tunnel: w1205 -> [w1223 w1227]
              tunnel: [w1223 w1225] -> w1204
              tunnel: w1202 -> [_ w1224]
              frame False {
              }
              frame True {
                w1226 = u16 0 items=["HOME", "TX1", "TX2", "TX3", "TX4", "TX5", "TX6", "TX7", "TX8", "TX9", "TX10", "TX11", "TX12", "RX8", "RX7", "RX6", "RX5", "RX4", "RX3", "RX2", "RX1"] ("Antenna Select")
                n641 = call "Gantry.vi"("COMPORT"=w1224, "error in (no error)"=w1227, "Antenna Select"=w1226) -> ("error out"=w1225:errorcluster)  [unwired: 16 in]
              }
            }
            n642 = property class="Arr (strict)"(reference=w1207, "Array Element.Value"=w1206) -> ()  [unwired: 1 in, 2 out]
            n643 = case shown="True" TRUE {
              tunnel: w1204 -> [w1228 _]
              tunnel: [w1228 w1231] -> w1209
              tunnel: w1202 -> [_ w1229]
              frame False {
              }
              frame True {
                w1233 = u32 15 items=["OFF"=0, "RED"=1, "AMBER"=2, "GREEN"=4, "GRE+AMBER"=6, "ALL"=7, "BUZZ"=8, "RED+BUZZ"=9, "ALL+BUZZ"=15] ("Select")
                n644 = call "RageATE-LightBar.vi"("VISA resource name"=w1229, "Select"=w1233) -> ("error out"=w1232:errorcluster)  [unwired: 11 in, 2 out]
                n645 = call "Time Delay2"("error in (no error)"=w1232, "Delay Time (s)"=3.0) -> ("error out"=w1231:errorcluster)  [unwired: 9 in]
              }
            }
            n646 = global read "Station References Global.vi" "Gantry"() -> (w1210:refnum<visa-resource-name>)
            n647 = call "RageATE-LightBar.vi"("VISA resource name"=w1210, "error in"=w1209, "Select"=w1208) -> ("error out"=w1200:errorcluster)  [unwired: 10 in, 2 out]
            n648 = Concatenate Strings("Sequence Complete!!" ("Text.Text"), "\r\n", "Start a new test by pressing the START button" ("string")) -> (w1214:string)
            n649 = control-ref of="Test Run 2"() -> (w1217:refnum<vi>)
            n650 = property class="VI"(error in=w1200, "Front Panel Window:State"=T5."Standard") -> (error out=w1220:errorcluster)  [unwired: 1 in, 1 out]
            n651 = control-ref of="Test Run"() -> (w1222:refnum<vi>)
            n652 = property class="Str"(reference=w1217, "Text.TextColor"=w1215, "Text.Text"=w1214) -> ()  [unwired: 1 in, 2 out]
            n653 = property class="Str"(reference=w1222, error in=w1220, "Text.TextColor"=w1215, "Text.Text"=w1214) -> (error out=w1221:errorcluster)  [unwired: 1 out]
          }
          frame True {
          }
        }
      }
      frame #12 {
        # "Get time Info"
        n654 = Get Date/Time In Seconds() -> (seconds since 1Jan1904=w1243:timestamp)
        n655 = Get Date/Time String(seconds (now)=w1243) -> (date string=w1246:string, time string=w1245:string)  [unwired: 2 in]
        n656 = local read "current time"() -> (w1238:timestamp)
        n657 = call <vilib>:"Space Constant.vi"() -> ("String"=w1244:string)
        n658 = Subtract(x=w1243, y=w1238) -> (x-y=w1242:dbl)
        n659 = Concatenate Strings(w1246, w1244, w1245) -> (w1239:string)
        "Seq End Time" <- w1239
        n660 = global write "Test Parameter Globals_1.0.0.vi" "Seq End Time"(w1239) -> ()
        n661 = Divide(x=w1242, y=60.0) -> (x/y=w1241:dbl)
        n662 = Number To Fractional String(number=w1241, precision (6)=i16 3) -> (F-format string=w1240:string)  [unwired: 2 in]
        "Total Test Time" <- w1240
        n663 = global write "Test Parameter Globals_1.0.0.vi" "Total Test Time"(w1240) -> ()
      }
      frame #13 {
        n664 = local read "ABORT AT SN SCAN(T)"() -> (w1248:bool)
        n665 = case shown="False" w1248 {
          tunnel: w1250 -> [w1255 w1389]
          tunnel: [w1254 w1389] -> w1249
          tunnel: [w1252 FALSE ("Stop Testing")] -> _
          frame False {
            n666 = flat-sequence {
              tunnel: [w1369] -> w1251
              tunnel: w1255 -> [w1368]
              frame #0 {
                w1359 = "/" ("string")
                n667 = local read "Results Archive File (Location on server)"() -> (w1357:path)
                n668 = Strip Path(path=w1357) -> (stripped path=w1360:path, name=w1364:string)
                n669 = Strip Path(path=w1360) -> (stripped path=w1361:path, name=w1363:string)
                n670 = Strip Path(path=w1361) -> (name=w1362:string)  [unwired: 1 out]
                n671 = Or(x="Send email notification", y="Send as attachment") -> (x .or. y?=w1366:bool)
                n672 = Concatenate Strings(w1362, w1359, w1363, w1359, w1364) -> (w1358:string)
                n673 = case shown="True" w1366 {
                  tunnel: [w1370 w1387] -> w1369
                  tunnel: w1368 -> [w1370 w1377]
                  tunnel: "Send as attachment" -> [_ w1376]
                  tunnel: w1357 -> [_ w1375]
                  tunnel: w1358 -> [_ w1371]
                  frame False {
                  }
                  frame True {
                    w1374 = "\r"
                    n674 = global read "Test Parameter Globals_1.0.0.vi" "Test Name"() -> (w1381:string)
                    n675 = Path To String(path=w1375) -> (string=w1378:string)
                    n676 = local read "result files array"() -> (w1384:path[])
                    n677 = Concatenate Strings(w1381, " has finished. The result file is attached" ("string")) -> (w1383:string)
                    n678 = Concatenate Strings(w1381, " has finished. The result file(local comp) is located at:" ("string"), w1374, w1378, w1374, w1374, "Also, a copy of the result has been archived on OneDrive." ("string"), w1374, w1371, w1374, "https://ragesystems.sharepoint.com/:f:/s/RageTestLab/EnRUXAqwPbJPm0PG5vQCj24BqplMiaAC4ONz4tBlZNFHJA?e=tcJCQL" ("string")) -> (w1379:string)
                    n679 = call "SendSMTP_Email_2.vi"("Send as attachment"=w1376, "message"=w1379, "message (attachment)"=w1383, "subject ([No Subject])"="RageAte Automated message. Test completed. <Do not reply>", "error in (no error)"=w1377, "file path"=w1384, "Recipient Email Address"="Recipient Email Address (use; to separate addresses)") -> ("error out"=w1387:errorcluster)  [unwired: 4 in]
                  }
                }
              }
            }
            n680 = flat-sequence {
              tunnel: w1251 -> [w1273]
              tunnel: [w1272] -> w1253
              frame #0 {
                n681 = local read "Send to Synology Drive"() -> (w1274:bool)
                n682 = global read "Sequence Globals.vi" "Stop Testing"() -> (w1276:bool)
                n683 = Not(x=w1276) -> (.not. x?=w1277:bool)
                n684 = And(x=w1277, y=w1274) -> (x .and. y?=w1275:bool)
                n685 = case shown="True" w1275 {
                  selector: w1275 -> [_ w1288]
                  tunnel: [w1279 w1283] -> w1272
                  tunnel: w1273 -> [w1279 w1289]
                  frame False {
                    n686 = local write "PostProcessMesssage"("Test Was Stopped or Data was not sent to Synology Drive!!" ("PostProcessMesssage")) -> ()
                  }
                  frame True {
                    n687 = flat-sequence {
                      tunnel: w1289 -> [w1294]
                      tunnel: w1288 -> [w1293]
                      tunnel: [w1292] -> w1287
                      tunnel: [w1291] -> w1286
                      tunnel: w1287 -> [w1310]
                      tunnel: w1286 -> [w1307]
                      tunnel: [w1303] -> w1285
                      tunnel: w1285 -> [w1321]
                      tunnel: [w1322] -> w1284
                      tunnel: [w1320] -> w1282
                      tunnel: [w1318] -> w1281
                      tunnel: [w1317] -> w1280
                      tunnel: w1284 -> [w1350]
                      tunnel: [w1348] -> w1283
                      tunnel: w1282 -> [w1347]
                      tunnel: w1281 -> [w1345]
                      tunnel: w1280 -> [w1344]
                      frame #0 {
                        n688 = case shown="False" FALSE {
                          tunnel: [TRUE ("OK") w1299] -> w1292
                          tunnel: [w1296 w1297] -> w1291
                          tunnel: w1294 -> [w1296 w1297]
                          tunnel: w1293 -> [_ _]
                          frame False {
                          }
                          frame True {
                            n689 = call "Display Message to User5"("Message"="Send To Synology Drive?") -> ("OK"=w1299:bool)  [unwired: 9 in, 1 out]
                          }
                        }
                      }
                      frame #1 {
                        n690 = local read "result files array"() -> (w1300:path[])
                        n691 = call "PostFinalTest.vi"("File Path"=w1300, "error in (no error)"=w1307, "Enable(t)"=w1310) -> ("ID"=→"ID":string[], "p/f(t = pass)"=w1311:bool, "error?(t)"=w1304:bool, "Output String"=→"db_out_str":string, "error out"=w1305:errorcluster)  [unwired: 7 in, 1 out]
                        "syn_error?(t)" <- w1304
                        n692 = Boolean To (0,1)(Boolean=w1311) -> (0, 1=w1312:i16)
                        n693 = Pick Line(multi-line string="There was an error sending the files to Syn Drive!!\nFiles Successfully Moved to Synology Drive" ("Message"), line index=w1312) -> (output string=w1306:string)  [unwired: 1 in]
                        n694 = case shown="False" FALSE {
                          tunnel: w1306 -> [_ w1316]
                          tunnel: w1305 -> [w1313 w1314]
                          tunnel: [w1313 w1314] -> w1303
                          tunnel: w1304 -> [_ w1315]
                          frame False {
                          }
                          frame True {
                            n695 = call "Display Message to User3"("Enable"=w1315, "Message"=w1316) -> ()  [unwired: 8 in, 2 out]
                          }
                        }
                      }
                      frame #2 {
                        n696 = local read "syn_error?(t)"() -> (w1319:bool)
                        n697 = case shown="False" w1319 {
                          tunnel: [w1332 FALSE ("pass?(t)")] -> w1323
                          tunnel: [w1329 w1337] -> w1322
                          tunnel: w1321 -> [w1328 w1341]
                          tunnel: [w1326 w1339] -> w1317
                          tunnel: [w1325 w1341] -> w1320
                          tunnel: [w1324 TRUE ("report_script_err?(t)")] -> w1318
                          frame False {
                            n698 = local read "Run Final Test Result"() -> (w1333:bool)
                            n699 = local read "ID"() -> (w1335:string[])
                            n700 = Index Array(array=w1335, index #1=1 ("index")) -> (element #1=w1327:string, element #2=w1331:string, element #3=w1334:string)  [unwired: 2 in]
                            n701 = call "FinalReportResult.vi"("TXID"=w1327, "RXID"=w1331, "BOUNCEID"=w1334, "error in (no error)"=w1328, "Run Final Report (T)"=w1333) -> ("standard output"=w1326:string, "result(ary)"=w1329:string[], "pass?(t)"=w1332:bool, "report_script_err?(t)"=w1324:bool, "error out"=w1325:errorcluster)  [unwired: 6 in]
                          }
                          frame True {
                            w1338 = "ERROR\n"
                            n702 = local read "db_out_str"() -> (w1340:string)
                            n703 = Concatenate Strings(w1338, w1340) -> (w1339:string)
                            n704 = Build Array(w1338) -> (w1337:string[])
                          }
                        }
                        "PASS" <- w1323
                        n705 = local write "PostProcessMesssage"(w1317) -> ()
                      }
                      frame #3 {
                        w1349 = TRUE  # Run Python (t)
                        n706 = Build Array(w1344) -> (w1343:string[])
                        n707 = local read "Place entry into DB log"() -> (w1355:bool)
                        n708 = local read "result files array"() -> (w1352:path[])
                        n709 = local read "Total Test Time"() -> (w1356:string)
                        n710 = global read "Tetra_Globals.vi" "Ver_Tags(ary)"() -> (w1354:string[])
                        n711 = local read "-ssid"() -> (w1353:string)
                        n712 = local read "ID"() -> (w1346:string[])
                        n713 = call "WAM_Database_log.vi"("log file path"="LogFilePath", "results file path in"=w1352, "Message_In(ary)"=w1350, "error in (no error)"=w1347, "-sid"=w1353, "Test Time"=w1356, "Ver_Tags(ary)"=w1354, "Enable(t)"=w1355, "-dbid(ary)"=w1346, "Run Python (t)"=w1349, "ProcessAsError(t)"=w1345, "Errors In"=w1343) -> ("error out"=w1348:errorcluster)  [unwired: 6 in, 1 out]
                      }
                    }
                  }
                }
              }
            }
            n714 = flat-sequence {
              tunnel: [w1258] -> w1254
              tunnel: w1253 -> [w1257]
              tunnel: [w1256] -> w1252
              frame #0 {
                n715 = local read "vis to run"() -> (w1259:path[])
                n716 = for {
                  tunnel: w1259 -> [w1260] mode=indexing
                  tunnel: w1257 -> [w1264]
                  tunnel: [w1261] -> w1258
                  n717 = Open VI Reference(vi path=w1260, error in (no error)=w1264) -> (vi reference=w1267:refnum<vi>, error out=w1263:errorcluster)  [unwired: 4 in]
                  n718 = property class="VI"(reference=w1267, error in=w1263) -> (error out=w1262:errorcluster, "FP.State"=w1266:T5)  [unwired: 1 out]
                  n719 = To Long Integer(number=w1266) -> (32bit integer=w1265:i32)
                  n720 = case shown="1, Default" w1265 {
                    tunnel: w1267 -> [_ w1271]
                    tunnel: w1262 -> [w1268 w1270]
                    tunnel: [w1268 w1269] -> w1261
                    frame 2 {
                    }
                    frame 1, Default {
                      n721 = invoke class="VI" method="FP.Close"(reference=w1271, error in=w1270) -> (error out=w1269:errorcluster)  [unwired: 1 in, 2 out]
                    }
                  }
                }
                n722 = global read "Sequence Globals.vi" "Stop Testing"() -> (w1256:bool)
              }
            }
          }
          frame True {
          }
        }
        n723 = local read "STOP TESTING"() -> (w1247:bool)
      }
      frame #14 {
        n724 = case shown="True" w1391 {
          tunnel: w1391 -> [_ w1396]
          tunnel: [FALSE ("OK") w1394] -> w1390
          frame False {
          }
          frame True {
            n725 = call "Display Message to User13"("Enable"=w1396, "Message"="QUIT or Restart the Test Sequence\n\nIf you QUIT the SW will close !!") -> ("QUIT (Close SW)"=w1394:bool)  [unwired: 8 in, 1 out]
            n726 = case shown="True" w1394 {
              frame False {
              }
              frame True {
                n727 = global read "Tetra_Globals.vi" "comport"() -> (w1397:refnum<visa-resource-name>)
                n728 = call "CloseComAndFt.vi"("ComPort"=w1397, "Skip(T)"=FALSE, "KillFT(t)"=TRUE) -> ("error out"=w1398:errorcluster)  [unwired: 11 in, 1 out]
                n729 = invoke class="VI" method="FP.Close"(error in=w1398) -> (reference out=w1401:refnum<vi>)  [unwired: 2 in, 2 out]
                n730 = invoke class="VI" method="Abort VI"(reference=w1401) -> ()  [unwired: 2 in, 3 out]
              }
            }
          }
        }
      }
    }
  }
  "error out" <- w1
